vi "PSHet_zi_OptimizeModulation.vi"(0 "zi Address":string="DEV1925", 1 "Stop Program":bool=TRUE) -> ()   [LabVIEW 2022 SP3]
doc: "Control a Zurich instrument device via the LabOne Labview API. \nRequirements: Zurich Instruments MFLI, HF2 or UHFLI \nThis example polls demod data for a given time from the instrument.\n\n© Zurich Instruments AG, www.zhinst.com"
uses:
  PSHet_DAQInAndOut_control.ctl
  zi_OptimizeModulation_Control.ctl
  <vilib>/DAQmx/read.llb/DAQmx Read (Analog 2D DBL NChan NSamp).vi
  <vilib>/Analysis/baseanly.llb/Mean (DBL).vi
  <vilib>/DAQmx/write.llb/DAQmx Write (Analog 1D DBL NChan 1Samp).vi
  <vilib>/Analysis/1siggen.llb/Ramp Pattern by Samples.vi
  <vilib>/DAQmx/create/channels.llb/DAQmx Create Channel (AI-Voltage-Basic).vi
  <vilib>/DAQmx/configure/timing.llb/DAQmx Timing (Sample Clock).vi
  <vilib>/DAQmx/create/channels.llb/DAQmx Create Channel (AO-Voltage-Basic).vi
  <vilib>/DAQmx/miscellaneous.llb/DAQmx Fill In Error Info.vi
  <instrlib>/Zurich Instruments LabOne/Public/Configure/ziGetValueDouble.vi
  <instrlib>/Zurich Instruments LabOne/Public/Configure/ziSetValueDouble.vi
  <vilib>/addons/Time Series Analysis/Statistical Analysis.llb/TSA Deviation and Variance (Array).vi
  <vilib>/addons/Time Series Analysis/Statistical Analysis.llb/TSA Mean (Array).vi
  <instrlib>/Zurich Instruments LabOne/Zurich Instruments LabOne.lvlib
  <vilib>/Analysis/NI_AALBase.lvlib
  <vilib>/addons/_Advanced Signal Processing/NI_AdvSigProcTSA.lvlib
panel:
  out "Acquistion time (ms)":dbl
  out "PSHet running":bool
  out "PSHet input error":errorcluster={"status"=TRUE, "code"=-50103, "source"="DAQmx Control Task.vi:3900001<append>\n<B>Task Name: </B>_unnamedTask<1C21>"}
  out "Status":string="Running PSHet..."
  in  "Pause PSHet":bool
  in  "Enable PSHet":bool
  in  "Amplify amplitude by":dbl=1.0
  out "Amplitude / Re / Im":T1(graph)={"[0]"=nan, "[1]"=nan, "[2]"=nan, "[3]"=0.0, "[4]"=0.0, "[5]"=0.0, "[6]"=0.0, "[7]"=0.0, "[8]"=0.0}
  out "Phase (1 = pi radians)":dbl(graph)=nan
  in  "Phase offset (rad)":dbl
  in  "Channels to read":tag="Dev1/ai4:7"
  in  "Sampling rate":dbl=100000.0
  in  "Target acquistion time (ms)":dbl=1.0
  in  "DAQ Input range (V)":dbl=10.0
  in  "DAQ Output range (V)":dbl=10.0
  in  "Channels to output":tag="Dev1/ao0:1"
  out "Samples per loop":i32=100
  out "PSHet output error":errorcluster
  in  "Cancel Button":bool
  in  "Optimization order":i32=7
  in  "Slow wiggler amp":dbl=0.005
  out "Slow wiggler osc address":string="demods/4/oscselect/"
  out "Slow wiggler amp address":string="sigouts/0/amplitudes/4"
  out "Slow wiggler enable address":string="sigouts/0/enables/4"
  out "Fast wiggler amp address":string="sigouts/0/amplitudes/7"
  in  "Fast wiggler\nsource":i32=8
  in  "Slow wiggler oscillator":i32=6
  in  "Slow wiggler source":i32=5
  in  "Keep mod2 activated?":bool=TRUE
  in  "Optimize PSHet":bool
  out "Optimal modulation":dbl=0.27257525083612044
  out "Phase leakage vs. modulation amplitude":dbl[](graph)=[0.25054863863248045, 0.20185890824577868, 0.18656755567836747, 0.18956495717052135, 0.19995883483514376, 0.21035859208104846, 0.21622410115159774, 0.215277174673977, 0.20697395311525213, 0.1920364400403578, 0.1720414170679394, 0.14906497041965316, 0.12538086095847767, 0.1032109696116823, 0.08452605007414782, 0.07089502068789777, 0.06338102739261942, 0.06248250964430646, 0.06811750119592652, 0.0796493976371142, 0.09595242258818182, 0.1155150244432459, 0.1365794355592982, 0.15731562578657687, 0.17602788223479315, 0.19139224717292969, 0.2027230459557554, 0.21026673687437203, 0.21552131482737735, 0.22157950070474897]
  out "Chart length needed:":dbl=30000.0
  out "Samples per acquisition:":dbl=1000.0
  in  "Sample rate":dbl=1000.0
  out "Waveform Chart":dbl[][](graph)=[[-0.14092939771744095, -0.665227293227987, 0.6799915049443154], [-0.14651752916434696, -0.6540510435502394, 0.6702612579595977], [-0.15210566053411873, -0.6438609333196119, 0.6615837312250977], [-0.15605022380758304, -0.6346569625992535, 0.6535603510970559], [-0.15966607344125233, -0.6267678446953842, 0.6467852705127449], [-0.1616383550460539, -0.6198648664205069, 0.6405930146703966], [-0.1626244958448666, -0.6139480278180354, 0.6351211754543004], [-0.1636106366412881, -0.6083599024023401, 0.6299763577096781], [-0.16492549103279835, -0.6027717769195728, 0.62492738189584], [-0.16722648620771996, -0.596526224829899, 0.6195225860282997], [-0.16952748136963997, -0.5889658195561722, 0.6128787021466868], [-0.17380075806445489, -0.5814054141589, 0.6068269597810081], [-0.17906017547355835, -0.5722014422037289, 0.5995640390322362], [-0.18596316072028496, -0.5606964770008249, 0.5907307647873227], [-0.19450971372166492, -0.5498489381165337, 0.583239130614505], [-0.2037136936779682, -0.5383439723517474, 0.5755983856469543], [-0.21423252766169015, -0.5268390062961934, 0.5687309684406832], [-0.2250800749266365, -0.5150053266202999, 0.5620422818403096], [-0.23527019482571027, -0.5044864999816006, 0.5566495245996471], [-0.2454603144747226, -0.49495381312809744, 0.5524762828502897], [-0.25367815271970184, -0.48837954621470475, 0.5503337045176875], [-0.2602524231991969, -0.48279141926249386, 0.5484695782762677], [-0.2641969854372826, -0.4791755723738725, 0.5471830372681302], [-0.2651831259909967, -0.47818943230826244, 0.5467972416551268], [-0.26386827191886186, -0.4785181456637076, 0.5464486075148144], [-0.2609098502414599, -0.48049042579130036, 0.5467586297719736], [-0.2549930068238768, -0.4824627059101911, 0.5457029376164886], [-0.24743259566829118, -0.48312013261455505, 0.5427964185002083], [-0.2392147573001126, -0.4841062726692899, 0.5399838732294739], [-0.23165434585792594, -0.48279141926249386, 0.5354916343588915], [-0.22475136137733348, -0.4795042857285921, 0.5295635320460162], [-0.22014937165967374, -0.47424487202404514, 0.5228517423546106], [-0.21653352255986602, -0.4666844647151091, 0.514471725169238], [-0.21554738189078948, -0.4571517770555433, 0.5054190549484804], [-0.21686223611570166, -0.4463042356765767, 0.496202277540073], [-0.21982065810645296, -0.43414184048071797, 0.4866212689416064], [-0.22475136137733348, -0.42197944494915735, 0.47810022631302285], [-0.23033949168000983, -0.41080318929877785, 0.4709729734978992], [-0.23527019482571027, -0.3992982199486827, 0.46345564299888964], [-0.24052961144992746, -0.3914090979332085, 0.45940785357799563], [-0.24381674680628107, -0.38516354290282123, 0.4558481773624323], [-0.24578902800763247, -0.3818764086402205, 0.45413856670061553], [-0.24611774154028299, -0.38089026835658285, 0.45348797032516663], [-0.2431593197370876, -0.3818764086402205, 0.45272071550897236], [-0.23954347083795613, -0.3848348294776816, 0.45329782748234193], [-0.2332979135744604, -0.3900942442500595, 0.45453430659876654], [-0.22770978331166813, -0.3946962321236938, 0.4556718787334672], [-0.21982065810645296, -0.3992982199486827, 0.45580718531473446], [-0.2132463869871169, -0.40291406749137787, 0.45586595326423074], [-0.2073295428901606, -0.40521506136658475, 0.4551755543890379], [-0.2033849801116484, -0.4058724881858455, 0.4539800951596721], [-0.20042655800294967, -0.40357149431410305, 0.4506004396090042], [-0.19911170372558423, -0.3992982199486827, 0.44618890507798536], [-0.20075527157163386, -0.3940388052875831, 0.44223213263654454], [-0.2040424072440254, -0.3874645368718301, 0.4379064640847843], [-0.2093018242652489, -0.379904128070702, 0.4337446255181976], [-0.21554738189078948, -0.3749734266076287, 0.43251097616342704], [-0.22343650717751085, -0.37168629226770866, 0.4336756536853347], [-0.23198305940175373, -0.37102886539672636, 0.4375826308332858], [-0.24052961144992746, -0.3743159997416429, 0.4449347835883802], [-0.24644645507267404, -0.3815476952125904, 0.45421855855956317], [-0.2523632986113858, -0.39502494554137685, 0.4687557381899311], [-0.2569652879723781, -0.4127754697283867, 0.48622499692243043], [-0.2582801420662071, -0.4334844137038221, 0.5045962432578016], [-0.25795142854313763, -0.45780920379725293, 0.5254790258125629], [-0.25532172034927364, -0.4841062726692899, 0.5473098428859704], [-0.25104844449892694, -0.5104033399960459, 0.5688030335401263], [-0.24513160094155323, -0.5360429791639318, 0.5894332678862912], [-0.23822861668502254, -0.5600390504090917, 0.6086021785951613], [-0.2300107781348794, -0.579104421187336, 0.6231106552587046], [-0.22212165297351055, -0.5945539452051685, 0.634690808566435], [-0.21390381410376091, -0.6057301963011648, 0.6423892218890226], [-0.20601468863485567, -0.6113183217484084, 0.6450985525007843], [-0.19812556301479944, -0.6129618880436634, 0.6441863200301476], [-0.19220871870035822, -0.6119757482672057, 0.6414503160897497], [-0.18596316072028496, -0.6096747554473569, 0.6374053691136222], [-0.18070374340001494, -0.6073737626161406, 0.6336850403735805], [-0.17544432601207816, -0.605401483037473, 0.6303107703298462], [-0.17084233574204577, -0.606716336090847, 0.6303108884997144], [-0.16656905901621227, -0.6106608952286836, 0.6329707579209672], [-0.16196706864592386, -0.6188787266586344, 0.6397219783908993], [-0.15769379182687798, -0.6307124036639074, 0.6501272707064689], [-0.15177694692626514, -0.6445183597927491, 0.6621481388089782], [-0.14586010193930504, -0.660296594873264, 0.6762150268509062], [-0.1402719704833164, -0.6767322558564977, 0.691117046396554], [-0.13468383895005748, -0.6921817766633975, 0.705163348749226], [-0.12909570733940656, -0.7050015914223215, 0.7167237581952113], [-0.12482243017308409, -0.7142055607818862, 0.725031187002382], [-0.12153529386041878, -0.7188075453957481, 0.7290096809861984], [-0.12054915296137905, -0.7181501190250259, 0.7281975636703029], [-0.12054915296137905, -0.7119045684584879, 0.7220389275321463], [-0.12252143475703947, -0.700399606676483, 0.7110352389351007], [-0.12547985743239393, -0.6829778068812071, 0.6944090144241486], [-0.13172541634230234, -0.661282734548313, 0.6742747513604876], [-0.1396145432481224, -0.6359718155703369, 0.6511162499018224], [-0.14783238361122814, -0.6083599024023401, 0.6260640418480861], [-0.15769379182687798, -0.5800905610336973, 0.6011425712600368], [-0.16755519980307576, -0.552478644536341, 0.5773278077918655], [-0.1787314618874738, -0.5258528663350106, 0.5553973104914895], [-0.18957901008877137, -0.503171646634506, 0.537700573779793], [-0.198454276585324, -0.48312013261455505, 0.5222922193872981], [-0.2073295428901606, -0.46832803153231345, 0.5121686094187875], [-0.2125889598694254, -0.4581379171677425, 0.5050588252918282], [-0.21554738189078948, -0.4532072165848266, 0.5018540176231927], [-0.21521866833390724, -0.4525497898362953, 0.5011191350171089], [-0.2122602463101868, -0.4561656369411528, 0.5031316929886138], [-0.20667211576303285, -0.46241119096196653, 0.5064952842434298], [-0.198454276585324, -0.47128645178799705, 0.511365837276919], [-0.188264155776651, -0.48049042579130036, 0.5160566263767962], [-0.1777453211276332, -0.4900231129520875, 0.5212638970905425], [-0.16722648620771996, -0.497254806525035, 0.5246208538569838], [-0.15736507822355128, -0.5028429332971325, 0.5268916239713523], [-0.14881852444358756, -0.5054726399894023, 0.5269246084549691], [-0.1429016794133996, -0.5044864999816006, 0.524335311268329], [-0.14060068410051235, -0.49988451324996525, 0.5192813100398346], [-0.13994325686585313, -0.4916666796834451, 0.5111949129766116], [-0.1429016794133996, -0.4811478524985639, 0.5019204577850457], [-0.14881852444358756, -0.46701317807903536, 0.4901512641185856], [-0.1567076510160994, -0.4525497898362953, 0.4789139799252666], [-0.16656905901621227, -0.43710026096461424, 0.4677626423271532], [-0.17807403471451122, -0.42197944494915735, 0.45801420698391426], [-0.19056515082009318, -0.4075160552296692, 0.44987155053085504], [-0.20141269870821388, -0.39535365895881186, 0.44370214204243624], [-0.2132463869871169, -0.38516354290282123, 0.44025558070797083], [-0.22310779362690247, -0.3779318474922087, 0.43887306698627404], [-0.23033949168000983, -0.3723437191376913, 0.4378311622174617], [-0.23592762190737826, -0.370042725088378, 0.4388547153326528], [-0.23789990314613924, -0.3713575788323425, 0.44102473317622665], [-0.23625633544782199, -0.37365857287465826, 0.4420834594530314], [-0.2326404864886279, -0.3776031340615869, 0.44351518892457137], [-0.22672364266923783, -0.38319126234824924, 0.4452405570983544], [-0.21784837678163893, -0.3894368174069938, 0.44622746443768246], [-0.20634340219907543, -0.3956823723759986, 0.4462534475387141], [-0.194838427295084, -0.40094178701725985, 0.4457760977524653], [-0.1826760249030404, -0.4058724881858455, 0.4450876393931262], [-0.17215719011021052, -0.40948833567409954, 0.44420580270836985], [-0.1613096414459182, -0.41080318929877785, 0.44133894090761827], [-0.15309180135608064, -0.41080318929877785, 0.43840205289265827], [-0.14553138832638368, -0.41014576248693274, 0.43519987531500065], [-0.1402719704833164, -0.408830908860278, 0.4322255634998852], [-0.13665612067650917, -0.4078447686376922, 0.43013050417691295], [-0.1336976980832168, -0.4078447686376922, 0.429199755099981], [-0.13139670271787868, -0.41014576248693274, 0.4306792773876148], [-0.13041056184299937, -0.4154051769540436, 0.4353945057995416], [-0.128438280086001, -0.42296558513992805, 0.4420365120713579], [-0.1258085710616461, -0.4344705538687981, 0.45231897896466106], [-0.12252143475703947, -0.44794780256925676, 0.4644014812654556], [-0.11759073024973879, -0.46438347116082607, 0.47904027818967854], [-0.11134517112023401, -0.48180527920486077, 0.4945038667204414], [-0.10444218460072047, -0.5011993666066632, 0.5119657947666927], [-0.09655305700399536, -0.5202647398477764, 0.5291482706630452], [-0.08800650193159876, -0.5370291191029919, 0.544192446793202], [-0.08077480134248968, -0.5534647844398692, 0.5593280219575893], [-0.07452924163692604, -0.5662846029925139, 0.5711679783088023], [-0.06992725021203366, -0.575488575065966, 0.5797214161592379], [-0.06795496815643756, -0.5827202672803569, 0.5866692318474125], [-0.06795496815643756, -0.5853499735120398, 0.5892813158311471], [-0.07025596388701183, -0.586336113345062, 0.590530217918005], [-0.07518666897898041, -0.585021260233898, 0.5898329510275032], [-0.08274708333437564, -0.5833776938396811, 0.5892169494083235], [-0.09129363851958627, -0.5833776938396811, 0.5904778252431242], [-0.09984019352155787, -0.5833776938396811, 0.5918594410095414], [-0.1087154619839723, -0.586336113345062, 0.5963296818765454], [-0.117262016613767, -0.5925816655720455, 0.6040723556929807], [-0.12547985743239393, -0.6017856371215244, 0.6147285154171823], [-0.13139670271787868, -0.614605454333125, 0.6284941988444742], [-0.13599869343542947, -0.6300549771714588, 0.6445656823588045], [-0.1396145432481224, -0.6468193524415049, 0.6617155698479744], [-0.1402719704833164, -0.6645698667836539, 0.6792122890084631], [-0.14060068410051235, -0.6810055276190861, 0.6953683060201132], [-0.1396145432481224, -0.6954689086855423, 0.7093442208368523], [-0.13764226153612147, -0.7069738705856179, 0.720248183511481], [-0.13599869343542947, -0.7142055607818862, 0.7270386699948721], [-0.1336976980832168, -0.7181501190250259, 0.7304893345753994], [-0.132054129966458, -0.7178214058393291, 0.7298670179713213], [-0.13073927546822722, -0.7138768475935018, 0.7257498960936838], [-0.12975313459173926, -0.7073025837787141, 0.7191055701052711], [-0.12909570733940656, -0.6994134670823502, 0.7112277410152218], [-0.1287669937128379, -0.6908669238482197, 0.7027645730522731], [-0.12810956645889582, -0.6833065200907678, 0.6952120981519532], [-0.12745213920388054, -0.67771839549742, 0.6895986306419428], [-0.12613728469062985, -0.6760748294280814, 0.6877410774232803], [-0.12449371654302638, -0.677389682284006, 0.6887346855818444], [-0.12219272112510132, -0.6833065200907678, 0.6941461384280053], [-0.1198917256940083, -0.6925104898666277, 0.7028120690947217], [-0.11660458934101617, -0.7043441650327582, 0.7139309021684664], [-0.11397488023924437, -0.7191362585807737, 0.7281121010744867], [-0.1116738847610535, -0.7349144911993433, 0.7433507690938476], [-0.11003031655426035, -0.7497065838135313, 0.7577378388165568], [-0.10937288926965574, -0.7621976838940085, 0.7700050248151523], [-0.10970160291209288, -0.7710729390207922, 0.7788375433757959], [-0.1116738847610535, -0.7766610625368955, 0.7846486236517366], [-0.1152897347922843, -0.7766610625368955, 0.7851714010389163], [-0.1195630120599196, -0.7717303653200991, 0.7809373026113774], [-0.1258085710616461, -0.7605541181121651, 0.7708893326087386], [-0.13238284359034563, -0.7451045994928283, 0.7567734677315491], [-0.1402719704833164, -0.7250530958729975, 0.7384972698245339], [-0.14816109722228138, -0.7017144594655083, 0.7171853967790203], [-0.1567076510160994, -0.6764035426424031, 0.6943191199917923], [-0.16459677743531914, -0.6484629186123119, 0.6690263492249687], [-0.17380075806445489, -0.6221658591901174, 0.6459853402713998], [-0.17971760264493414, -0.5968549380998718, 0.6233251429508072], [-0.18760672861900846, -0.5735162953514401, 0.6034212671565087], [-0.19352357299982798, -0.5528073578377533, 0.5857024399694588], [-0.19812556301479944, -0.5360429791639318, 0.5714856203185472], [-0.20009784443400264, -0.5235518730839088, 0.560487030319885], [-0.20042655800294967, -0.5156627532770801, 0.5532439608980911], [-0.19812556301479944, -0.5110607666595257, 0.5481211963959736], [-0.194838427295084, -0.5110607666595257, 0.5469416056302939], [-0.18563444713974858, -0.5140191866333361, 0.5465124629796438], [-0.17610175318927423, -0.5189498865466406, 0.5480153394049361], [-0.16393935023956402, -0.526181579655643, 0.5511289915490549], [-0.15046209249218567, -0.5340706992793982, 0.554860660982478], [-0.1369848342966476, -0.5419598187662475, 0.5590038371822003], [-0.12317886202010969, -0.548205371596469, 0.5618737949894014], [-0.11003031655426035, -0.553793497740573, 0.5646183743917379], [-0.09885405256912966, -0.5564232041377004, 0.5651361834214876], [-0.09129363851958627, -0.5554370642405482, 0.5628897412160784], [-0.0866916472888084, -0.5518212179328075, 0.558589382525746], [-0.08570550630386592, -0.54491823853859, 0.5516170052697811], [-0.08833521559161803, -0.5347281259085266, 0.541975349025454], [-0.09392334777045852, -0.5215795931450926, 0.5299687417591823], [-0.10312733001207844, -0.5071162066642754, 0.5174959838075888], [-0.11397488023924437, -0.48969439960509303, 0.50278313250361], [-0.12646599831934513, -0.47161516514852736, 0.488277086016722], [-0.1402719704833164, -0.4525497898362953, 0.4737906056309553], [-0.15309180135608064, -0.43545669403156745, 0.46158382989371693], [-0.16854134058755144, -0.4186923109639196, 0.4513418158639376], [-0.18234731131986343, -0.40291406749137787, 0.4422559075106061], [-0.19319485942535564, -0.39042295767121954, 0.4356080113876762], [-0.2037136936779682, -0.3822051220676013, 0.4331050961679291], [-0.2122602463101868, -0.3766169937682243, 0.4323132801090846], [-0.21850580389095609, -0.3749734266076287, 0.43399292274863155], [-0.22179293942185763, -0.3779318474922087, 0.4382061037072189], [-0.22245036652490235, -0.3848348294776816, 0.44450198148734915], [-0.22047808521263307, -0.3946962321236938, 0.45210142856627855], [-0.21554738189078948, -0.4078447686376922, 0.46130036759697746], [-0.2089731107033897, -0.42263687174325054, 0.4714781928721327], [-0.20009784443400264, -0.4374289743504884, 0.4810231334857551], [-0.1902364372432495, -0.45189236308678876, 0.49030256971707475], [-0.18004631623022538, -0.4647121845264523, 0.49837143822195684], [-0.16919876777587567, -0.4755597254559905, 0.5047625931986757], [-0.1590086462375248, -0.48312013261455505, 0.5086146007693798], [-0.1498046652735464, -0.4867359794712938, 0.5092674655322084], [-0.14224425218248232, -0.4867359794712938, 0.5070950019383285], [-0.1369848342966476, -0.4821339925576467, 0.5012165516090394], [-0.13336898446040085, -0.47424487202404514, 0.4926413347021356], [-0.13304027083731707, -0.4627399043290507, 0.4814851324007063], [-0.1343551253280451, -0.44827651594706014, 0.4679777072164331], [-0.13895711601185873, -0.4301972798046227, 0.4520827132744958], [-0.14520267471319537, -0.41211804291950466, 0.4369497660414395], [-0.154735369387356, -0.38910810398508827, 0.4187459266981731], [-0.1655829182269603, -0.36642687727184187, 0.4021024237625902], [-0.17906017547355835, -0.34144465516461636, 0.3855476611018478], [-0.19319485942535564, -0.31744857203224575, 0.37161519020849354], [-0.2083156835788848, -0.29246634705880625, 0.35907100716551893], [-0.22409393427794427, -0.2668266935753615, 0.3484459438485796], [-0.23987218437553975, -0.2428306062021015, 0.3413288270064119], [-0.2569652879723781, -0.21883451744522248, 0.33751993311241724], [-0.2727435368257259, -0.19516714086823977, 0.3353792625594037], [-0.2878643580870167, -0.17281461729270303, 0.3357540477892614], [-0.3003554708937939, -0.1514482333181451, 0.3363777285597547], [-0.31284658333191384, -0.13238284359034563, 0.3397031085808872], [-0.32270798762880853, -0.1149610211544283, 0.3425733230482259], [-0.33125453783479286, -0.09885405256912966, 0.3456901684246783], [-0.33750009364637984, -0.08504807897921357, 0.3480509861347468], [-0.34144465516461636, -0.07321438694954918, 0.34920595498485146], [-0.3434169359101129, -0.06433911769566525, 0.34939192024966353], [-0.34210208208079046, -0.0577648440459419, 0.3469446811404721], [-0.3398010878697672, -0.05349156611494882, 0.3439856493560555], [-0.3358565263363857, -0.052505425047378484, 0.33993591446351945], [-0.3296109705007827, -0.05546384824269451, 0.33424486583395185], [-0.3220505606827909, -0.062038121930698104, 0.3279714807857356], [-0.31350401029215486, -0.07321438694954918, 0.3219396075751815], [-0.3039713192689968, -0.08932135657004811, 0.31682308577129925], [-0.2937812010415308, -0.11035903019615817, 0.3138256038490819], [-0.28293365556150724, -0.13599869343542947, 0.31392212101975475], [-0.2720861098020284, -0.1662403454200604, 0.31885216573293407], [-0.2602524231991969, -0.1987829901555856, 0.3274843522311402], [-0.25104844449892694, -0.23494148128448594, 0.34383545645188957], [-0.24052961144992746, -0.27307225033718857, 0.3638996398575702], [-0.2309969187694889, -0.31087430244508535, 0.38730144384150733], [-0.2214642258699434, -0.3467040704657786, 0.4114001893749113], [-0.21390381410376091, -0.3795754146415767, 0.4356975293577658], [-0.20601468863485567, -0.40850219545299654, 0.4575107601174367], [-0.20075527157163386, -0.43282698692594507, 0.4771183078390439], [-0.19681070873007078, -0.45090622296069977, 0.49198666341224845], [-0.19352357299982798, -0.46372604442884496, 0.5024870322587865], [-0.19286614585061995, -0.47030031170495185, 0.5083106662318306], [-0.19352357299982798, -0.47227259186886067, 0.5103849276155705], [-0.19516714086823977, -0.4696428849817093, 0.5085810184116454], [-0.19812556301479944, -0.46372604442884496, 0.5042772878105402], [-0.20174141227610976, -0.4568230636843234, 0.4993865325988384], [-0.20535726150562883, -0.4502487962087541, 0.4948692588356276], [-0.20995925138818072, -0.44400324201656344, 0.4911433254811718], [-0.21423252766169015, -0.44071610819576196, 0.4900267991972841], [-0.21686223611570166, -0.43841511450664145, 0.48911863804293315], [-0.21850580389095609, -0.4410448215789429, 0.49220455196557716], [-0.21883451744522248, -0.4456468089177948, 0.4964772143050443], [-0.21817709033642824, -0.4538646433323827, 0.5035815298587717], [-0.21653352255986602, -0.46241119096196653, 0.5105985467263379], [-0.2125889598694254, -0.47325873194754303, 0.5188139292877173], [-0.20765825645333097, -0.48279141926249386, 0.5255563775530943], [-0.20174141227610976, -0.49068053964535335, 0.5305346260271939], [-0.19549585444113232, -0.4975835198664926, 0.5346101274259557], [-0.18925029651113684, -0.5002132265895001, 0.5348167413092374], [-0.18234731131986343, -0.5002132265895001, 0.5324131985597856], [-0.17610175318927423, -0.4975835198664926, 0.5278268529727], [-0.17084233574204577, -0.4913379663376554, 0.5201923690776528], [-0.1655829182269603, -0.4824627059101911, 0.5100862333005467], [-0.16098092784551665, -0.4735874453066194, 0.5001998875270302], [-0.1567076510160994, -0.46339733106248987, 0.48917724223723086], [-0.15177694692626514, -0.4532072165848266, 0.477946673576482], [-0.14684624277646752, -0.44498938215803535, 0.4685929675645541], [-0.14191553856662292, -0.43775768773611773, 0.46018671564781943], [-0.1363274070561032, -0.4318408467572898, 0.4528484060286549], [-0.12975313459173926, -0.4265814324871455, 0.44587845258452113], [-0.1241650029127001, -0.4232942985363594, 0.44112924537112636], [-0.11824815752087511, -0.4200071645609699, 0.4363354730475479], [-0.11298873932163633, -0.41672003056095214, 0.431766185665591], [-0.1087154619839723, -0.4131041831324574, 0.42716989336319505], [-0.1060857528304466, -0.4078447686376922, 0.4214161153287037], [-0.10444218460072047, -0.40159921384295644, 0.4149579478494798], [-0.10509961189342096, -0.39502494554137685, 0.4087672149526127], [-0.10542832553936615, -0.3868071100247859, 0.40091753789496587], [-0.10772932105342398, -0.37826056092258104, 0.3933022483588129], [-0.1106877438377864, -0.3697140116517618, 0.38592774848090217], [-0.11331745296110843, -0.3614961756550187, 0.37884077151066664], [-0.11594716206718864, -0.35525062019272474, 0.3736933870685304], [-0.117262016613767, -0.3499912049962634, 0.3691127525771276], [-0.11791944388544148, -0.3463753570113456, 0.36589736701838793], [-0.11660458934101617, -0.3434169359101129, 0.3626731615728928], [-0.11430359387790834, -0.3434169359101129, 0.36193991689684685], [-0.10937288926965574, -0.3440743628232617, 0.36103960455804], [-0.10641446647558184, -0.3453892166465354, 0.36141077688828], [-0.10148376177019686, -0.3473614973738892, 0.3618825275705647], [-0.09622434335075086, -0.34834763773416705, 0.36139341577878487], [-0.09227977949069568, -0.3486763511870896, 0.36068096093361246], [-0.08997878388764544, -0.3490050646397605, 0.3604174200758102], [-0.08932135657004811, -0.3476902108275669, 0.35898020480916715], [-0.09096492486200772, -0.34473178973540247, 0.3565313792772306], [-0.09589562969723567, -0.34111594170615106, 0.35433890201486995], [-0.10312733001207844, -0.3358565263363857, 0.3513329652596856], [-0.11266002568189482, -0.33026839743514586, 0.34895486202519754], [-0.1258085710616461, -0.32468026846077536, 0.34820263250058064], [-0.13994325686585313, -0.3187634259374788, 0.34812962651521157], [-0.15572151020292557, -0.31350401029215486, 0.3500485012239638], [-0.1741294716545091, -0.3089020215490944, 0.354600524274564], [-0.19155129154904277, -0.306601027158851, 0.3615191380120406], [-0.2089731107033897, -0.30725845412876585, 0.37158783434155923], [-0.2250800749266365, -0.3102168754807733, 0.38326955261543266], [-0.24020089791286348, -0.31679114507810524, 0.39755892765481066], [-0.2523632986113858, -0.32698126275320416, 0.4130423473176805], [-0.26189599080291753, -0.34111594170615106, 0.43005766553418867], [-0.26847026115328043, -0.3582090412124717, 0.44764941453113605], [-0.27307225033718857, -0.37727442063071553, 0.4657300101630324], [-0.27307225033718857, -0.3986407931195172, 0.48320072003586034], [-0.2710999692645514, -0.42165073155174165, 0.5012828869544218], [-0.2671554070914608, -0.4420309617270178, 0.516491415866243], [-0.2609098502414599, -0.461753764227069, 0.5303682576577228], [-0.2533494391930111, -0.47687457888406243, 0.5399956502836528], [-0.24480288740812445, -0.4929815330641953, 0.5504173376863043], [-0.23559890836667435, -0.502185506621665, 0.5547045417917784], [-0.22573750202445986, -0.5090884866662126, 0.5568918270870363], [-0.217519663226588, -0.5123756199836123, 0.556635949111984], [-0.20634340219907543, -0.5150053266202999, 0.5548045476367071], [-0.1974681358729612, -0.5153340399488096, 0.5518721205271231], [-0.1885928693550767, -0.5182924598946399, 0.5515381621929872], [-0.18004631623022538, -0.5225657331155742, 0.5527129647608168], [-0.17084233574204577, -0.5294687128488675, 0.5563490105748679], [-0.1616383550460539, -0.5413023921475639, 0.564920558633397], [-0.15309180135608064, -0.5560944908388858, 0.5767826127613499], [-0.1429016794133996, -0.575488575065966, 0.5929654205859107], [-0.1336976980832168, -0.598169791177434, 0.6129291749868054], [-0.12383628928210527, -0.6234807121962402, 0.6356599916810025], [-0.11331745296110843, -0.6487916318457858, 0.6586132603422973], [-0.10279861636424256, -0.6760748294280814, 0.6838455458015443], [-0.09326592045936613, -0.6997421802806196, 0.7059303441438171], [-0.08373322432665023, -0.7201223981345077, 0.724974152057252], [-0.07715895099860967, -0.7355719175473041, 0.7396076997999844], [-0.07058467756171738, -0.7470768784927337, 0.7504039306166636], [-0.0672975408023899, -0.7520075759576037, 0.7550128166433205], [-0.06565397241249496, -0.7510214364686147, 0.753885695665412], [-0.06598268609101984, -0.744775886325401, 0.7476930090054158], [-0.06894110918546298, -0.7335996385007506, 0.7368319388735493], [-0.07452924163692604, -0.7194649717655752, 0.7233149061485014], [-0.08208965600483406, -0.7036867386422951, 0.7084587057578033], [-0.08997878388764544, -0.6859362257591042, 0.6918126100025529], [-0.09786791161426697, -0.6695005650939518, 0.6766159433422027], [-0.10838674834072598, -0.6550371832383053, 0.6639438219011071], [-0.117262016613767, -0.6432035068455573, 0.6538051175684925], [-0.12515114380287323, -0.6339995361123312, 0.6462338745267217], [-0.131067989093187, -0.6303836904177982, 0.6438652148623143], [-0.13599869343542947, -0.6287401241837955, 0.6432804896581261], [-0.13895711601185873, -0.6300549771714588, 0.6451963688280186], [-0.13994325686585313, -0.6346569625992535, 0.6499027429684633], [-0.14060068410051235, -0.6382728082608786, 0.6535753438852787], [-0.14060068410051235, -0.642874793608186, 0.6580703249853315], [-0.1396145432481224, -0.6455044995007344, 0.6604303744998979], [-0.1396145432481224, -0.6468193524415049, 0.6617155698479744], [-0.1392858296301243, -0.6445183597927491, 0.6593970415809337], [-0.14092939771744095, -0.6402450877009507, 0.6555721680076105], [-0.14454524748601766, -0.6330133963802218, 0.6493067753901987], [-0.14881852444358756, -0.6228232856936409, 0.6403559935065724], [-0.15407794217564486, -0.6113183217484084, 0.6304364383269513], [-0.16065221424484938, -0.598169791177434, 0.619367607337539], [-0.16788391339816627, -0.5846925469555224, 0.608317666062082], [-0.17544432601207816, -0.5718727289162142, 0.5981798472097754], [-0.18201859773642226, -0.5593816238164158, 0.5882504322016462], [-0.1885928693550767, -0.548534084900955, 0.580049060571353], [-0.19352357299982798, -0.5393301122858216, 0.5729994269847543], [-0.19615328158612783, -0.5320984193863076, 0.5671021405270956], [-0.19681070873007078, -0.526181579655643, 0.5617842199988716], [-0.19615328158612783, -0.522237019792319, 0.5578598522196858], [-0.19319485942535564, -0.5179637465682814, 0.5528206729740067], [-0.18957901008877137, -0.5156627532770801, 0.5494072043425872], [-0.18563444713974858, -0.5113894799909064, 0.5440398406461147], [-0.18070374340001494, -0.5081023466663224, 0.5392789978912604], [-0.1770878939530834, -0.5025142199595187, 0.5328045264881504], [-0.1744581852442985, -0.4942963864410928, 0.5241799080921131], [-0.17380075806445489, -0.4854211260722226, 0.5155971035033108], [-0.17478689883382315, -0.4739161586654533, 0.5051207632320851], [-0.17807403471451122, -0.4601101973855695, 0.49336776909086055], [-0.18300473848595328, -0.4463042356765767, 0.4823672927253313], [-0.18957901008877137, -0.4321695601470869, 0.4719223768629382], [-0.19516714086823977, -0.41672003056095214, 0.4601584474345812], [-0.20108398514005532, -0.40390020772509433, 0.4511874852876355], [-0.2073295428901606, -0.39272395161238255, 0.4440919291375243], [-0.21160281919092377, -0.38450611605229307, 0.43888575548901815], [-0.21390381410376091, -0.3795754146415767, 0.4356975293577658], [-0.21521866833390724, -0.3776031340615869, 0.43462995991136316], [-0.2145612412193576, -0.3776031340615869, 0.43430479284337187], [-0.21193153275068627, -0.38089026835658285, 0.4358811433209802], [-0.2102879649492535, -0.38549225632771184, 0.4391187856276804], [-0.20700082932672786, -0.39042295767121954, 0.44190432133969454], [-0.20437112080982006, -0.39535365895881186, 0.44505288525430614], [-0.20305626654506598, -0.3992982199486827, 0.4479630741896116], [-0.2033849801116484, -0.40225664066766237, 0.45075032456588254], [-0.2040424072440254, -0.40422892113583814, 0.4528071605403125], [-0.20667211576303285, -0.40422892113583814, 0.4539982203892567], [-0.2109453920706127, -0.40521506136658475, 0.45683389146838654], [-0.21521866833390724, -0.40521506136658475, 0.4588227557104654], [-0.21949194455297083, -0.4065299150041169, 0.46199922674924354], [-0.22442264782776938, -0.40915962226731223, 0.4666659633527569], [-0.22770978331166813, -0.4134328965362813, 0.4719941793647739], [-0.22968206458948842, -0.41902102436355165, 0.47784146916395825], [-0.23033949168000983, -0.4269101458808718, 0.48508613058242817], [-0.22968206458948842, -0.43578540741866695, 0.4926081324066255], [-0.2270523562169754, -0.4453180955380373, 0.4998609593450011], [-0.22343650717751085, -0.4558369235692022, 0.5076526111709863], [-0.21982065810645296, -0.4647121845264523, 0.5140802818409801], [-0.2145612412193576, -0.47293001858822453, 0.5193258406005326], [-0.2106166785100641, -0.4795042857285921, 0.5237210567646665], [-0.20700082932672786, -0.48312013261455505, 0.5255990923502992], [-0.20469983437535216, -0.4841062726692899, 0.5256052753074777], [-0.20272755297822093, -0.4811478524985639, 0.5221127432849318], [-0.20272755297822093, -0.47588843881337156, 0.5172700135642558], [-0.20469983437535216, -0.4666844647151091, 0.5096041716859513], [-0.20700082932672786, -0.4561656369411528, 0.5009355564020992], [-0.21160281919092377, -0.4426883884911778, 0.4906615558554213], [-0.21653352255986602, -0.42986856641335275, 0.48132499496956843], [-0.22245036652490235, -0.41737745736292714, 0.4729567712611856], [-0.2290246374979244, -0.40521506136658475, 0.46545840903283797], [-0.23461276774300144, -0.3973259394582111, 0.4614228569916986], [-0.23954347083795613, -0.3933813784504793, 0.46057570857861574], [-0.2428306062021015, -0.3946962321236938, 0.46341322700277005], [-0.2444741738744362, -0.39962693336289373, 0.46847551436613927], [-0.24348803327181412, -0.4114606161096351, 0.47810695556109256], [-0.24085832498673154, -0.4265814324871455, 0.48988207893144964], [-0.23559890836667435, -0.4456468089177948, 0.5040911861183274], [-0.2290246374979244, -0.4653696112569759, 0.5186724974996502], [-0.2208067987653311, -0.4867359794712938, 0.5344787704791213], [-0.2122602463101868, -0.5054726399894023, 0.5482307925878636], [-0.2033849801116484, -0.5225657331155742, 0.5607498511472233], [-0.19385228657403697, -0.5367004057902094, 0.5706365170450959], [-0.1853057335589483, -0.5452469518454433, 0.5758753800837183], [-0.1777453211276332, -0.550506364722904, 0.5784899798468358], [-0.17084233574204577, -0.5514925046306862, 0.5773483232379093], [-0.16492549103279835, -0.550506364722904, 0.5746804983578586], [-0.15999478704271725, -0.5459043784584396, 0.5688672273043507], [-0.1567076510160994, -0.5409736788378665, 0.5632138218140236], [-0.15374922856938977, -0.5370291191029919, 0.5586046008136863], [-0.1511195197097585, -0.5350568392227344, 0.5559882466710345], [-0.14816109722228138, -0.5350568392227344, 0.555191437190032], [-0.14520267471319537, -0.5393301122858216, 0.5585344991691229], [-0.14092939771744095, -0.5465618050704886, 0.5644385723025238], [-0.13599869343542947, -0.5583954839256335, 0.5747183319546075], [-0.1300818482175034, -0.5731875820648644, 0.5877629551690438], [-0.12383628928210527, -0.5896232461066138, 0.6024873433462828], [-0.11660458934101617, -0.6103321819684733, 0.6213710667562375], [-0.1087154619839723, -0.6307124036639074, 0.6400134278356135], [-0.10279861636424256, -0.6501064847773921, 0.6581838626675833], [-0.09688177065696921, -0.6671995725555206, 0.6741968162961756], [-0.09195106583393023, -0.6826490936714198, 0.6888140413772114], [-0.08997878388764544, -0.6931679162724105, 0.6989835060281001], [-0.09030749754603731, -0.6984273274861903, 0.7042415607535029], [-0.09326592045936613, -0.6990847538838554, 0.7052786860752163], [-0.09951147987101891, -0.6934966294749632, 0.7005998213811181], [-0.10937288926965574, -0.6842926597180914, 0.692978263043836], [-0.12054915296137905, -0.670486704749867, 0.6812374912804208], [-0.13468383895005748, -0.653064903860116, 0.6668084471031749], [-0.15013337888299938, -0.6323559698909977, 0.6499339228810962], [-0.1655829182269603, -0.6113183217484084, 0.633346503356454], [-0.18037502981525233, -0.5896232461066138, 0.6165960782636828], [-0.19450971372166492, -0.567270742866339, 0.5996916911582252], [-0.20535726150562883, -0.5475479449867868, 0.5847908659617937], [-0.21291767342840207, -0.5288112862121277, 0.5700660594031963], [-0.21916323099922735, -0.5110607666595257, 0.5560716042387372], [-0.22179293942185763, -0.4959399531567997, 0.5432757542119439], [-0.22212165297351055, -0.48180527920486077, 0.5305415683896583], [-0.2211355123177679, -0.46832803153231345, 0.5179112471524182], [-0.21982065810645296, -0.4558369235692022, 0.5060715587932094], [-0.21883451744522248, -0.4423596751092201, 0.4935287511262319], [-0.21784837678163893, -0.42986856641335275, 0.4819179387164022], [-0.2171909496712756, -0.4163913171595948, 0.46963138483816524], [-0.21850580389095609, -0.40225664066766237, 0.4577719861407705], [-0.22212165297351055, -0.38812196371787927, 0.4471875305058354], [-0.22606621557298007, -0.3730011460066744, 0.4361602787345284], [-0.23132563231383774, -0.3588664681029879, 0.42696216471030507], [-0.23757118960699586, -0.3450605031910949, 0.4189353422591305], [-0.24381674680628107, -0.33191196476662593, 0.41183996695129055], [-0.24907616332246757, -0.3204069933133073, 0.40583195598611294], [-0.2540068662461338, -0.31153172940837925, 0.40195958320253655], [-0.2569652879723781, -0.3036426057816176, 0.3977813359982819], [-0.25795142854313763, -0.29969804391316635, 0.39542111351421744], [-0.2549930068238768, -0.2973970494729249, 0.3917479273260843], [-0.24973359038232373, -0.29904061693151734, 0.3896051292527201], [-0.24151575205956038, -0.30134161136282056, 0.3861821140752588], [-0.23033949168000983, -0.3069297406439358, 0.38374750438166894], [-0.21817709033642824, -0.31284658333191384, 0.3814108381392984], [-0.2040424072440254, -0.3197495663637374, 0.3793060626245444], [-0.19089386439667327, -0.32599512234368355, 0.3777741220043648], [-0.17741660754049055, -0.3309258243684969, 0.37548442559598355], [-0.16459677743531914, -0.3351990994106198, 0.373430763847574], [-0.1544066557816336, -0.33651395326114103, 0.37024729045478416], [-0.14553138832638368, -0.3355278128736291, 0.36572981584766334], [-0.1382996887745252, -0.33289810516247864, 0.3604829431968997], [-0.13402641170576485, -0.32698126275320416, 0.35338339693087323], [-0.13139670271787868, -0.3204069933133073, 0.34630295241190817], [-0.13041056184299937, -0.31284658333191384, 0.3389393741403599], [-0.12975313459173926, -0.30594360018791694, 0.3323211736142101], [-0.13041056184299937, -0.30068418438372474, 0.3277466908737791], [-0.13139670271787868, -0.2973970494729249, 0.3251308944415032], [-0.13271155721396527, -0.29805447645712824, 0.3262649664832073], [-0.132054129966458, -0.30134161136282056, 0.32900617012442085], [-0.13139670271787868, -0.3089020215490944, 0.3356866878537899], [-0.12975313459173926, -0.3187634259374788, 0.344159843171426], [-0.12810956645889582, -0.3355278128736291, 0.35915313479078437], [-0.1241650029127001, -0.35360705295074235, 0.3747731258305749], [-0.1198917256940083, -0.3730011460066744, 0.391795713111029], [-0.11627587570423698, -0.3946962321236938, 0.4114671249607044], [-0.11266002568189482, -0.4163913171595948, 0.43136296826749915], [-0.11003031655426035, -0.43677154757849485, 0.45041764545268886], [-0.10772932105342398, -0.4558369235692022, 0.4683939661264504], [-0.10740060740936822, -0.4739161586654533, 0.48593355092658536], [-0.10772932105342398, -0.48969439960509303, 0.5014042397300049], [-0.10970160291209288, -0.5038290733085331, 0.5156337622697119], [-0.11298873932163633, -0.516320179932904, 0.5285385354157623], [-0.117262016613767, -0.5284825728934006, 0.5413355802017413], [-0.12153529386041878, -0.540644965527932, 0.5541369924526218], [-0.12679471194779196, -0.5531360711389295, 0.567482521469106], [-0.131067989093187, -0.5669420295752992, 0.5818952505940319], [-0.13501255257180217, -0.5817341274396153, 0.5971959346645657], [-0.1382996887745252, -0.5984985044462423, 0.6142696995127785], [-0.13994325686585313, -0.6169064471286443, 0.6325801764607463], [-0.14060068410051235, -0.635643102327911, 0.6510074545706702], [-0.1402719704833164, -0.6543797567798233, 0.6692451656803305], [-0.1386284023933257, -0.6734451237053358, 0.6875653922301652], [-0.13501255257180217, -0.6905382106438607, 0.7036131108152964], [-0.13238284359034563, -0.7050015914223215, 0.7173231218809777], [-0.12909570733940656, -0.7165065530943033, 0.7280435030137563], [-0.1258085710616461, -0.7247243826919954, 0.7355632042325574], [-0.12285014838870895, -0.7286689408492888, 0.7389523559185343], [-0.12120658022767436, -0.7289976540276133, 0.7390051519903305], [-0.11890558479093533, -0.7263679485947732, 0.7360359602901568], [-0.11824815752087511, -0.7214372508696887, 0.7310638369523524], [-0.11759073024973879, -0.7145342739700464, 0.7241455713588036], [-0.117262016613767, -0.7076312969715859, 0.7172812788537117], [-0.11791944388544148, -0.7013857462685895, 0.7112291897236769], [-0.11759073024973879, -0.6977699010876239, 0.7076089419336781], [-0.117262016613767, -0.6954689086855423, 0.7052853206246296], [-0.1156184484298711, -0.6977699010876239, 0.7072838613181862], [-0.11298873932163633, -0.7030293122509328, 0.7120510298409183], [-0.10904417562694887, -0.7115758552685341, 0.7198825112747959], [-0.10279861636424256, -0.7240669563293214, 0.7313279105670795], [-0.09523820238939307, -0.7365580570675769, 0.7426897647238225], [-0.0866916472888084, -0.7500352969776343, 0.7550287335075236], [-0.07551538264959917, -0.764169962824945, 0.7678921181393863], [-0.06401040401577515, -0.7746887836561054, 0.7773287871582004], [-0.052176711357640404, -0.7832353254158497, 0.7849713269842221], [-0.04132915944241505, -0.7875085962402038, 0.7885923462552961], [-0.031139034643375835, -0.7881660225175937, 0.7887809065448563], [-0.022921191870621138, -0.784550177981127, 0.7848849360301088], [-0.016675631247889122, -0.7773184888287366, 0.7774973374568599], [-0.01273106659260495, -0.7664709549010125, 0.7665766789848588], [-0.010758784250008285, -0.7536511417681602, 0.7537279316351423], [-0.011087497974467092, -0.7405026151286573, 0.7405856166735311], [-0.013059780315401476, -0.7273540881337612, 0.7274713240992953], [-0.015032062646365224, -0.7145342739700464, 0.7146923754912359], [-0.01799048612412768, -0.7036867386422951, 0.7039166738556576], [-0.020948909579486336, -0.6941540558793919, 0.6944700930251637], [-0.022592478156122725, -0.686264938966628, 0.6866367209260691], [-0.02456476043897063, -0.6800193879849667, 0.6804629273449603], [-0.023907333012459286, -0.6750886897837547, 0.6755118797221225], [-0.023578619298789433, -0.670486704749867, 0.6709011645051547], [-0.022921191870621138, -0.665556006449812, 0.6659505828199207], [-0.022592478156122725, -0.6606253080985085, 0.6610115110718452], [-0.022592478156122725, -0.653064903860116, 0.6534555751717613], [-0.02522218786437755, -0.6435322200826994, 0.6440263015166646], [-0.028838038684383893, -0.6313698301554347, 0.6320280807888716], [-0.03574102652085526, -0.6169064471286443, 0.6179409239447176], [-0.04363015532819994, -0.6004707840542041, 0.6020537791232885], [-0.05447770718005396, -0.5820628407200967, 0.5846066807065622], [-0.0672975408023899, -0.5633261833583318, 0.5673317793453089], [-0.08241836966974073, -0.5409736788378665, 0.5472159618052028], [-0.09819662526615838, -0.5199360265228508, 0.5291276300572791], [-0.11266002568189482, -0.5008706532678491, 0.5133845466038174], [-0.12745213920388054, -0.4814765658518331, 0.49805996752612025], [-0.14060068410051235, -0.4656983246218734, 0.48646015450923813], [-0.1511195197097585, -0.4525497898362953, 0.47711468382159766], [-0.15933735983952152, -0.4433458152543596, 0.4711092295255761], [-0.16393935023956402, -0.4361141208055213, 0.46590947288388895], [-0.16656905901621227, -0.4321695601470869, 0.463158482745672], [-0.16656905901621227, -0.42921113963007645, 0.46039923306201913], [-0.16328192304274658, -0.42953985302183745, 0.45952744393187134], [-0.15933735983952152, -0.42986856641335275, 0.4584488833347729], [-0.15374922856938977, -0.42953985302183745, 0.45622725764656386], [-0.14816109722228138, -0.42921113963007645, 0.4540637764815195], [-0.1429016794133996, -0.42625271909317336, 0.4495689830420842], [-0.13895711601185873, -0.422308158346327, 0.4445821191818218], [-0.13534126619327902, -0.41507646355169997, 0.4365841601906621], [-0.1336976980832168, -0.4058724881858455, 0.427326047812347], [-0.13304027083731707, -0.3940388052875831, 0.4158921659961059], [-0.13402641170576485, -0.3792467012122018, 0.4022326931206118], [-0.13566997981448808, -0.3637971697498838, 0.38827145676818603], [-0.13764226153612147, -0.34933377809217975, 0.37547234342483116], [-0.1392858296301243, -0.3332268186272572, 0.3611656891070842], [-0.1392858296301243, -0.3194208528885718, 0.34846839683939007], [-0.13895711601185873, -0.307587167613341, 0.3375188080251687], [-0.13599869343542947, -0.29871190344030973, 0.3282140244917588], [-0.13172541634230234, -0.29509605502016273, 0.32316136371635734], [-0.12646599831934513, -0.2941099145365725, 0.32014729509964407], [-0.1195630120599196, -0.29673962248769936, 0.3199214238011934], [-0.11134517112023401, -0.3026564653179497, 0.322488268206069], [-0.10378475730693973, -0.31087430244508535, 0.3277409156177769], [-0.09622434335075086, -0.3200782798386492, 0.334229306730801], [-0.08965007022898236, -0.32895354356540724, 0.3409509772918971], [-0.08406193799019845, -0.33782880710762103, 0.3481303094107524], [-0.07978866034287696, -0.3450605031910949, 0.3541651891163255], [-0.07748766466759524, -0.3509773453505023, 0.35942931867743266], [-0.07584409631994568, -0.3545931932966854, 0.36261365070682283], [-0.07485795530808936, -0.3582090412124717, 0.3659473058778629], [-0.07485795530808936, -0.3611674622118925, 0.36884366503098126], [-0.07518666897898041, -0.3637971697498838, 0.3714854181662862], [-0.07485795530808936, -0.36839915790279604, 0.3759277231282593], [-0.07321438694954918, -0.3756308534726159, 0.3826994702595813], [-0.07091339123615026, -0.3848348294776816, 0.39131388300918685], [-0.06631139976927175, -0.3976546528739095, 0.40314566187871803], [-0.06006583983578334, -0.4131041831324574, 0.4174481659280741], [-0.05184799766762835, -0.4324982735366388, 0.43559496263652503], [-0.04198658683972736, -0.45353592995872644, 0.4554752608407802], [-0.029495466102617218, -0.4762171521705106, 0.47712970829953766], [-0.016346917528137828, -0.4979122332077099, 0.49818050312167034], [-0.002212227316732457, -0.5192785998722829, 0.5192833121091216], [0.011265035921287303, -0.539658825596705, 0.5397763880337141], [0.023427444611510473, -0.5570806307346219, 0.5575730214964759], [0.03460371239416328, -0.570886589052261, 0.5719343620304546], [0.040849273943313294, -0.5820628407200967, 0.5834944847458667], [0.04643740804696267, -0.5889658195561722, 0.5907936775826175], [0.04775226314199056, -0.5942252319335644, 0.5961408431752351], [0.04676612182029741, -0.5968549380998718, 0.598684296841259], [0.0428215565588506, -0.5994846442512705, 0.6010120834053132], [0.036575994977682005, -0.600799497321383, 0.6019118202778826], [0.02901557846235757, -0.6040866299803822, 0.6047830688061302], [0.019154165838942444, -0.6086886156639422, 0.6089899119918752], [0.008306612243586142, -0.6142767410756962, 0.6143329019623995], [-0.0028696547797994465, -0.6218371459380092, 0.6218437673458537], [-0.013388494037921028, -0.6293975506780882, 0.6295399340567523], [-0.023907333012459286, -0.6379440950200623, 0.6383919085818169], [-0.03311131688319169, -0.6464906392066561, 0.6473380151725757], [-0.042315300537971334, -0.653064903860116, 0.6544343766287353], [-0.04987571552180023, -0.6573381758357935, 0.659227627159193], [-0.05710741667495384, -0.6599678816477914, 0.6624340433929705], [-0.06269554929348325, -0.6593104551961617, 0.6622846882060475], [-0.0672975408023899, -0.6550371832383053, 0.6584851330309762], [-0.07058467756171738, -0.6484629186123119, 0.6522931499883234], [-0.07255695960422626, -0.6392589479819486, 0.6433634392487632], [-0.07354310062180197, -0.6284114109363035, 0.6327001572972969], [-0.07485795530808936, -0.6165777338728362, 0.621105317462884], [-0.07551538264959917, -0.6034292034504425, 0.6081359852808834], [-0.07551538264959917, -0.5915955257523353, 0.5963957068146093], [-0.07650152365982202, -0.5804192743153491, 0.5854391660275479], [-0.07683023732935193, -0.5702291624751175, 0.5753817716135596], [-0.07683023732935193, -0.5623400434760335, 0.5675642781788789], [-0.07781637833630875, -0.555765777539835, 0.5611871240698925], [-0.07847380567291956, -0.548534084900955, 0.5541189226825947], [-0.08077480134248968, -0.5432746720007695, 0.549246700280905], [-0.08241836966974073, -0.5376865457278444, 0.5439665514677895], [-0.0853767926416755, -0.5311122794365519, 0.5379307112352572], [-0.08965007022898236, -0.5235518730839088, 0.5311720050056581], [-0.09425206142559839, -0.5156627532770801, 0.5242056144303241], [-0.09951147987101891, -0.5058013533248564, 0.5154973750189], [-0.10509961189342096, -0.49528252647123877, 0.5063108822135676], [-0.1106877438377864, -0.48476369937123903, 0.49724000328210566], [-0.1156184484298711, -0.47325873194754303, 0.4871770242754959], [-0.12054915296137905, -0.4627399043290507, 0.47818439679496544], [-0.12383628928210527, -0.45189236308678876, 0.46855323535253], [-0.12613728469062985, -0.44301710187289106, 0.46062432321902036], [-0.12646599831934513, -0.4344705538687981, 0.45250227724285413], [-0.12613728469062985, -0.42789628606057645, 0.44610071308344673], [-0.1241650029127001, -0.4213220181540797, 0.43923705550617825], [-0.12252143475703947, -0.41672003056095214, 0.43435824597403966], [-0.12022043932782811, -0.41080318929877785, 0.42803295944380676], [-0.11824815752087511, -0.40521506136658475, 0.4221159470043826], [-0.11791944388544148, -0.3986407931195172, 0.4157156205691693], [-0.11890558479093533, -0.39272395161238255, 0.4103299163655013], [-0.12186400749289447, -0.38450611605229307, 0.403355661425308], [-0.12712342557597045, -0.3746447131747607, 0.39562485569029665], [-0.13402641170576485, -0.3641258831910051, 0.3880086826919633], [-0.14224425218248232, -0.3526209126025377, 0.38023010833388793], [-0.15342051496286835, -0.34144465516461636, 0.37432914253629185], [-0.1642680638375743, -0.3292822570332215, 0.367982066945983], [-0.17511561242308304, -0.317777285508935, 0.36283313092899694], [-0.18464830639655566, -0.3085733080655381, 0.35960044981288025], [-0.19220871870035822, -0.2993693304224695, 0.3557614194119862], [-0.19812556301479944, -0.29213763356248545, 0.352984611085838], [-0.20272755297822093, -0.28885049858519735, 0.352892435834851], [-0.20469983437535216, -0.28490593657863494, 0.35081820775302663], [-0.20437112080982006, -0.28293365556150724, 0.34902579914736914], [-0.2033849801116484, -0.28096137453514125, 0.3468497428508367], [-0.20108398514005532, -0.2799752340184922, 0.34470407706250805], [-0.19779684944401188, -0.27833166648560687, 0.341455868625262], [-0.19648199515823084, -0.27570195841962686, 0.33855094786128825], [-0.19418100014798262, -0.27241482331400585, 0.33453863271627066], [-0.19385228657403697, -0.26847026115328043, 0.33114194861674223], [-0.19319485942535564, -0.2628821313620513, 0.3262380552569515], [-0.19418100014798262, -0.25795142854313763, 0.3228702530520832], [-0.1958245680137617, -0.2530207256660615, 0.31994804117912135], [-0.1974681358729612, -0.24907616332246757, 0.31785625653836486], [-0.1987829901555856, -0.24743259566829118, 0.31739181869472266], [-0.198454276585324, -0.2487474497921507, 0.31821281192482304], [-0.1974681358729612, -0.2530207256660615, 0.32095662059182173], [-0.19516714086823977, -0.2602524231991969, 0.3253022235640839], [-0.19056515082009318, -0.2710999692645514, 0.3313763269189964], [-0.18399087923310697, -0.28457722307642164, 0.33887584678589766], [-0.17577303960080853, -0.29904061693151734, 0.34687382724167865], [-0.16689777261209882, -0.31580500464498895, 0.3571941593331298], [-0.15736507822355128, -0.3322406782321631, 0.3676243138265914], [-0.14816109722228138, -0.3463753570113456, 0.37673279479605626], [-0.1396145432481224, -0.36018132188100965, 0.3862936775541807], [-0.13073927546822722, -0.3713575788323425, 0.39369938977115077], [-0.12449371654302638, -0.38056155492820515, 0.40040702110236365], [-0.11824815752087511, -0.3874645368718301, 0.40510664532982354], [-0.11331745296110843, -0.39272395161238255, 0.4087455777322099], [-0.11003031655426035, -0.3973259394582111, 0.41227972631137316], [-0.10707189376504267, -0.40225664066766237, 0.41626289216751644], [-0.10444218460072047, -0.40817348204546794, 0.42132382008295344], [-0.10246990271613649, -0.41573389035614056, 0.42817607190653], [-0.10049762082182453, -0.42460915211962486, 0.43634012404842387], [-0.09885405256912966, -0.4361141208055213, 0.44717742572195335], [-0.09753919796210497, -0.44926265607900545, 0.4597290824890823], [-0.09589562969723567, -0.46306861769589186, 0.4728937687153568], [-0.09523820238939307, -0.47818943230826244, 0.48758122232676404], [-0.09359463411504779, -0.4916666796834451, 0.500495833595119], [-0.09425206142559839, -0.5054726399894023, 0.5141848314184605], [-0.09458077508046742, -0.5173063199148471, 0.5258814996162767], [-0.09688177065696921, -0.5274964329357907, 0.5363194609983986], [-0.09852533891777929, -0.535714265850437, 0.544699015094149], [-0.10115504812100973, -0.5422885320752335, 0.551642271567975], [-0.10345604365964414, -0.548534084900955, 0.5582049760328497], [-0.1060857528304466, -0.5560944908388858, 0.5661230163974631], [-0.1087154619839723, -0.5633261833583318, 0.5737206990613581], [-0.11003031655426035, -0.5731875820648644, 0.5836528718291347], [-0.1106877438377864, -0.585021260233898, 0.5954004127992839], [-0.11200259840160343, -0.6001420707867922, 0.6105039616390461], [-0.11101645747914501, -0.6162490206167963, 0.6261689143053809], [-0.10970160291209288, -0.6346569625992535, 0.6440682431677507], [-0.10707189376504267, -0.6524074773988899, 0.6611353167093826], [-0.10444218460072047, -0.6698292783128177, 0.677922880576575], [-0.10016890717182642, -0.6842926597180914, 0.6915853194711825], [-0.09655305700399536, -0.6971124746881563, 0.7037672166154532], [-0.09227977949069568, -0.7050015914223215, 0.7110153314879064], [-0.08899264291084263, -0.7096035761241, 0.7151621674420202], [-0.08439065165347506, -0.7096035761241, 0.7146040983192089], [-0.08044608767622402, -0.7073025837787141, 0.7118627101081048], [-0.07650152365982202, -0.702700599054914, 0.7068526119598125], [-0.07288567327702397, -0.6964550482877871, 0.700258492026044], [-0.06992725021203366, -0.6911956370523529, 0.6947238508950332], [-0.06696882712495675, -0.686922365380997, 0.690179078114598], [-0.06401040401577515, -0.68396394650921, 0.6869526999340757], [-0.06105198088447078, -0.681334240830006, 0.68406409940686], [-0.05940841246862469, -0.6803481011965664, 0.6829369650808306], [-0.05875098510037216, -0.6803481011965664, 0.6828800898049653], [-0.05907969878463515, -0.6803481011965664, 0.682908448922882], [-0.06006583983578334, -0.6790332483488073, 0.6816847199976768], [-0.06269554929348325, -0.6760748294280814, 0.6789756305548977], [-0.06664011344725074, -0.6714728444037357, 0.6747715802343085], [-0.07255695960422626, -0.663583727115445, 0.6675386695012018], [-0.07978866034287696, -0.6537223303204269, 0.6585735459907879], [-0.08734907461074631, -0.6432035068455573, 0.6491075504519852], [-0.09556691604344972, -0.6303836904177982, 0.6375865687001399], [-0.10345604365964414, -0.6159203073605253, 0.624548619395472], [-0.1116738847610535, -0.6021143503877731, 0.6123828438815991], [-0.11759073024973879, -0.5886371062806011, 0.6002676259228599], [-0.12186400749289447, -0.5771321414882868, 0.5898579024316655], [-0.12515114380287323, -0.5656271764087875, 0.5793072686298222], [-0.12613728469062985, -0.5560944908388858, 0.57022074438807], [-0.12482243017308409, -0.5498489381165337, 0.5638390673075023], [-0.12285014838870895, -0.5442608119241725, 0.5579533944295771], [-0.1195630120599196, -0.5399875389073514, 0.5530658695201313], [-0.1149610211544283, -0.5367004057902094, 0.5488746322797623], [-0.1106877438377864, -0.5327558460182888, 0.5441328588704804], [-0.10641446647558184, -0.5301261394846553, 0.5407011766587778], [-0.10378475730693973, -0.5255241530141397, 0.5356742585289023], [-0.10246990271613649, -0.5202647398477764, 0.5302598235690962], [-0.10312733001207844, -0.5143478999625632, 0.5245846055607418], [-0.10575703918504134, -0.5067874933297802, 0.5177046597556066], [-0.10970160291209288, -0.4979122332077099, 0.5098539336509736], [-0.1156184484298711, -0.48969439960509303, 0.5031582560407046], [-0.12252143475703947, -0.480819139145053, 0.4961839845693463], [-0.13073927546822722, -0.47325873194754303, 0.4909853210784956], [-0.1386284023933257, -0.4666844647151091, 0.48683901195010426], [-0.14553138832638368, -0.46241119096196653, 0.4847715900453212], [-0.1511195197097585, -0.4607676241228989, 0.48491639761629957], [-0.15605022380758304, -0.4604389107543559, 0.4861642344795167], [-0.15802250542993873, -0.46306861769589186, 0.4892889298943305], [-0.15966607344125233, -0.4676706048061598, 0.49417512038538186], [-0.15802250542993873, -0.47424487202404514, 0.49987929629407335], [-0.15637893741197428, -0.48312013261455505, 0.5077986161891379], [-0.15276308774902642, -0.4919953930289939, 0.5151660195901617], [-0.15046209249218567, -0.49988451324996525, 0.5220377073203446], [-0.14750366999990816, -0.5071162066642754, 0.5281327292688892], [-0.14618881555195945, -0.5120469066529498, 0.5325065299180279], [-0.14586010193930504, -0.5153340399488096, 0.5355785115813607], [-0.14750366999990816, -0.516320179932904, 0.5369765924780969], [-0.1514482333181451, -0.5156627532770801, 0.5374426876351432], [-0.1567076510160994, -0.5120469066529498, 0.5354897968214132], [-0.16459677743531914, -0.5081023466663224, 0.5340974572397023], [-0.17281461729270303, -0.503171646634506, 0.532021238229174], [-0.18201859773642226, -0.4979122332077099, 0.5301390024322135], [-0.19089386439667327, -0.4942963864410928, 0.5298767640810622], [-0.1997691308647927, -0.4916666796834451, 0.5307012620650322], [-0.20667211576303285, -0.4919953930289939, 0.5336411061712943], [-0.21193153275068627, -0.4946250997847155, 0.5381161249313153], [-0.21488995477676326, -0.5008706532678491, 0.5450221132843338], [-0.21521866833390724, -0.5090884866662126, 0.5527116449429259], [-0.2132463869871169, -0.5209221664969119, 0.562880027280144], [-0.2093018242652489, -0.5340706992793982, 0.5736190072422169], [-0.20305626654506598, -0.5488627982052046, 0.5852198036950458], [-0.1958245680137617, -0.5636548966519603, 0.5967026931039514], [-0.1879354421979616, -0.5781182813388661, 0.6078984106348262], [-0.18004631623022538, -0.5906093859305248, 0.6174432141803049], [-0.17314333088355183, -0.6021143503877731, 0.6265144084315548], [-0.1662403454200604, -0.6083599024023401, 0.6306644300231032], [-0.1603235006439162, -0.6136193145601432, 0.6342178553620039], [-0.15605022380758304, -0.6159203073605253, 0.6353813794639254], [-0.15309180135608064, -0.6142767410756962, 0.6330663585036149], [-0.1524343741417058, -0.6109896084886619, 0.6297178257768331], [-0.1511195197097585, -0.6057301963011648, 0.6242965480830049], [-0.15046209249218567, -0.6011282105883295, 0.619672467390842], [-0.1498046652735464, -0.5955400850185826, 0.6140923632497475], [-0.1491472380538405, -0.5912668124786318, 0.6097879485179504], [-0.14783238361122814, -0.5886371062806011, 0.6069168448268485], [-0.14553138832638368, -0.5869935398992416, 0.6047650790775269], [-0.1429016794133996, -0.5869935398992416, 0.604137654729957], [-0.1392858296301243, -0.5866648266222687, 0.6029727698092914], [-0.13468383895005748, -0.586336113345062, 0.601605995886775], [-0.13041056184299937, -0.5860074000676216, 0.6003428916662713], [-0.12515114380287323, -0.5837064071189924, 0.5969723431675292], [-0.12153529386041878, -0.5794331344696906, 0.5920418777207478], [-0.117262016613767, -0.5735162953514401, 0.5853813471353249], [-0.11430359387790834, -0.5662846029925139, 0.5777054294013472], [-0.11233131204188385, -0.5564232041377004, 0.5676487521063673], [-0.1106877438377864, -0.5452469518454433, 0.556368596465191], [-0.11003031655426035, -0.5343994125940812, 0.545609203314909], [-0.1106877438377864, -0.5225657331155742, 0.5341598281998722], [-0.11200259840160343, -0.5136904733038699, 0.5257589603723979], [-0.11331745296110843, -0.5058013533248564, 0.5183395163122808], [-0.11463230751630296, -0.502185506621665, 0.5151027557559468], [-0.11693330297752613, -0.5028429332971325, 0.5162600245148741], [-0.11824815752087511, -0.5087597733331555, 0.5223209106661205], [-0.1195630120599196, -0.5186211732207597, 0.5322247975862434], [-0.12022043932782811, -0.5337419859644774, 0.5471137556427186], [-0.11923429842556194, -0.5541222110410402, 0.5668052952205431], [-0.11759073024973879, -0.5781182813388661, 0.5899562077467032], [-0.1152897347922843, -0.6050727697735487, 0.615958423653666], [-0.11200259840160343, -0.6323559698909977, 0.6421982985850206], [-0.10772932105342398, -0.6599678816477914, 0.6687026330300374], [-0.10279861636424256, -0.6865936521739255, 0.6942466411383869], [-0.09852533891777929, -0.7089461497408267, 0.7157596563380797], [-0.09392334777045852, -0.7280115144919712, 0.7340452033010665], [-0.08997878388764544, -0.7411600414690598, 0.7466018943321253], [-0.08702036094991306, -0.7503640101415157, 0.755393070484175], [-0.08636293362743236, -0.7533224286064912, 0.7582567096612587], [-0.08570550630386592, -0.7526650022824899, 0.7575289033902948], [-0.0876777882713082, -0.7470768784927337, 0.7522042654323327], [-0.09030749754603731, -0.738530336102118, 0.7440312503222798], [-0.09392334777045852, -0.7283402276707416, 0.7343712157348476], [-0.09819662526615838, -0.7184788322104989, 0.725158196222193], [-0.10214118906776018, -0.7082887233566553, 0.7156156357559388], [-0.1060857528304466, -0.6980986142870198, 0.7061132077953647], [-0.1087154619839723, -0.6898807842344648, 0.6983942641018386], [-0.11200259840160343, -0.6816629540406993, 0.6908031303925912], [-0.1136461666003111, -0.6741025501373847, 0.6836151689983707], [-0.1152897347922843, -0.6668708593348343, 0.6767632274129968], [-0.11660458934101617, -0.6589817419700044, 0.6692186238481476], [-0.11824815752087511, -0.6504351980097214, 0.6610964933858197], [-0.1198917256940083, -0.6409025141791371, 0.6520199832605028], [-0.12186400749289447, -0.6307124036639074, 0.642377593365251], [-0.12515114380287323, -0.6185500134042146, 0.6310839309295725], [-0.12679471194779196, -0.606387622827852, 0.6195020969268279], [-0.13271155721396527, -0.5912668124786318, 0.6059775581296696], [-0.1382996887745252, -0.5784469946219237, 0.5947501403970128], [-0.1442165338720282, -0.5639836099453535, 0.5821305016309096], [-0.1491472380538405, -0.5511637913283285, 0.5709872358385135], [-0.154735369387356, -0.5393301122858216, 0.5610882324177531], [-0.1586799326352621, -0.5288112862121277, 0.5521056940898691], [-0.1613096414459182, -0.5202647398477764, 0.5446982650534928], [-0.16196706864592386, -0.5130330466442197, 0.5379927864523868], [-0.1603235006439162, -0.5077736333325464, 0.5324825701996782], [-0.1567076510160994, -0.5038290733085331, 0.5276372077459273], [-0.1507908061011054, -0.5015280799452373, 0.5237062938118822], [-0.1442165338720282, -0.498898373229919, 0.5193245569521254], [-0.13566997981448808, -0.49659737984139835, 0.5147963685654802], [-0.12679471194779196, -0.49528252647123877, 0.5112550048710104], [-0.1195630120599196, -0.492652819719369, 0.506953759854176], [-0.11298873932163633, -0.4880508328665049, 0.5009591507051067], [-0.1067431801204472, -0.4834488459663749, 0.49509281268106275], [-0.10345604365964414, -0.47687457888406243, 0.48796774171614876], [-0.10148376177019686, -0.46832803153231345, 0.4791973487217575], [-0.10148376177019686, -0.45912405727775113, 0.4702061823011409], [-0.10345604365964414, -0.44794780256925676, 0.45973947709146323], [-0.10509961189342096, -0.43578540741866695, 0.4482798788025191], [-0.1067431801204472, -0.4239517253284841, 0.43718322464525633], [-0.10740060740936822, -0.41047447589297886, 0.42429257103031737], [-0.10740060740936822, -0.3986407931195172, 0.4128551470078325], [-0.10509961189342096, -0.3871358234484324, 0.4011484441166929], [-0.10049762082182453, -0.3769457071995947, 0.3901125965244519], [-0.09392334777045852, -0.36839915790279604, 0.38018355408920534], [-0.08504807897921357, -0.3637971697498838, 0.37360615152333926], [-0.07485795530808936, -0.362153602540519, 0.36980933642349284], [-0.06269554929348325, -0.3628110294250167, 0.368188233073318], [-0.05020442921345694, -0.36708430414982757, 0.37050151290623917], [-0.03672716763043671, -0.3743159997416429, 0.3761134835455116], [-0.023578619298789433, -0.38450611605229307, 0.38522837975629043], [-0.010430070525272339, -0.39633979920962775, 0.3964770142248983], [0.003047192427820339, -0.4098170490806396, 0.40982837761538127], [0.014880887113591354, -0.42362301193254476, 0.4238842967604349], [0.027372009674298106, -0.4361141208055213, 0.43697225687631785], [0.038548277571306064, -0.44827651594706014, 0.44993088852994895], [0.048738404466217605, -0.45780920379725293, 0.46039624146096947], [0.056627535151335326, -0.4647121845264523, 0.46814964721193925], [0.06155824191206011, -0.4676706048061598, 0.47170458101131796], [0.06780380390026441, -0.46931417161972416, 0.47418682763912096], [0.06878994527615954, -0.4666844647151091, 0.4717270886619984], [0.06813251769194636, -0.4604389107543559, 0.4654525008029295], [0.06451666599900902, -0.45287850321068285, 0.45745091415579897], [0.05892853163176645, -0.4433458152543596, 0.44724499297793024], [0.05169682845410899, -0.4334844137038221, 0.4365561808019215], [0.042164129019213736, -0.4249378655148263, 0.4270245933482585], [0.03164528853782095, -0.4183635975640411, 0.4195587253929644], [0.021126448343487966, -0.4154051769540436, 0.41594204867965723], [0.010607608435402774, -0.4170487439620629, 0.4171836240758416], [0.0004174825466486398, -0.4242804387241775, 0.42428064412091354], [-0.009115215623556744, -0.4361141208055213, 0.4362093689065341], [-0.016346917528137828, -0.45287850321068285, 0.4531734330066362], [-0.022921191870621138, -0.4749022987405021, 0.4754551234194274], [-0.02752318384460778, -0.5002132265895001, 0.5009698570812645], [-0.030810320935775404, -0.5278251462552324, 0.5287236148457177], [-0.034097457999380715, -0.5570806307346219, 0.558123163631204], [-0.03705588133308016, -0.5837064071189924, 0.5848814478619869], [-0.03837073614090267, -0.6100034687080311, 0.611209084706555], [-0.04100044574334666, -0.6313698301554347, 0.6326996909922239], [-0.04428758272166619, -0.6484629186123119, 0.6499734969970131], [-0.047574719672524995, -0.6616114477728732, 0.6633197281673723], [-0.051519283977342234, -0.6685144254359896, 0.6704966619138005], [-0.05710741667495384, -0.671801557621237, 0.674224435823567], [-0.06335297665517553, -0.6695005650939518, 0.6724913429273213], [-0.0695985365367828, -0.665556006449812, 0.6691851418026884], [-0.07650152365982202, -0.6589817419700044, 0.6634074308990635], [-0.08307579699873885, -0.6517500509367491, 0.6570233762531061], [-0.08932135657004811, -0.6448470730289735, 0.651003880428948], [-0.09490948873506563, -0.6389302347418218, 0.645940907451441], [-0.09852533891777929, -0.6349856758423693, 0.6425838863011224], [-0.10148376177019686, -0.6330133963802218, 0.6410966494217966], [-0.10312733001207844, -0.633670822868525, 0.642007755366159], [-0.10312733001207844, -0.6353143890852553, 0.6436300328404442], [-0.10214118906776018, -0.6386015215014651, 0.6467184285051433], [-0.09984019352155787, -0.6425460803705849, 0.65025651064947], [-0.09753919796210497, -0.6461619259715781, 0.6534823101770926], [-0.09556691604344972, -0.6487916318457858, 0.6557923581402679], [-0.09523820238939307, -0.6497777715448341, 0.6567202354032755], [-0.09556691604344972, -0.6497777715448341, 0.6567679863055342], [-0.09655305700399536, -0.6471480656761246, 0.6543111734680728], [-0.10016890717182642, -0.6418886538946944, 0.6496574897303508], [-0.10641446647558184, -0.6346569625992535, 0.6435165101619329], [-0.11200259840160343, -0.627425271192444, 0.6373437478940408], [-0.11923429842556194, -0.6178925868946805, 0.6292917184108149], [-0.12679471194779196, -0.6093460421864507, 0.6223981829232917], [-0.1343551253280451, -0.6001420707867922, 0.6149974022954681]] caption="Signals vs time"
  in  "Update\nmodulation":bool=TRUE
  out "Present modulation":dbl=0.27257525083612044
  in  "N voltages":dbl=30.0
  in  "Ending V":dbl=0.4
  in  "Starting V":dbl=0.1
  out "PSHet Optimization Errors":errorcluster
  in  "time":dbl=1.0 caption="recording time [s]"
  # "Input / Output settings"
  # "Amplitude / Phase"
  # "Should be sidebands:\n+1,+2,-1,-2\n(Im,Re,Im,Re)\n(Negative sidebands can be supplied as zero)"
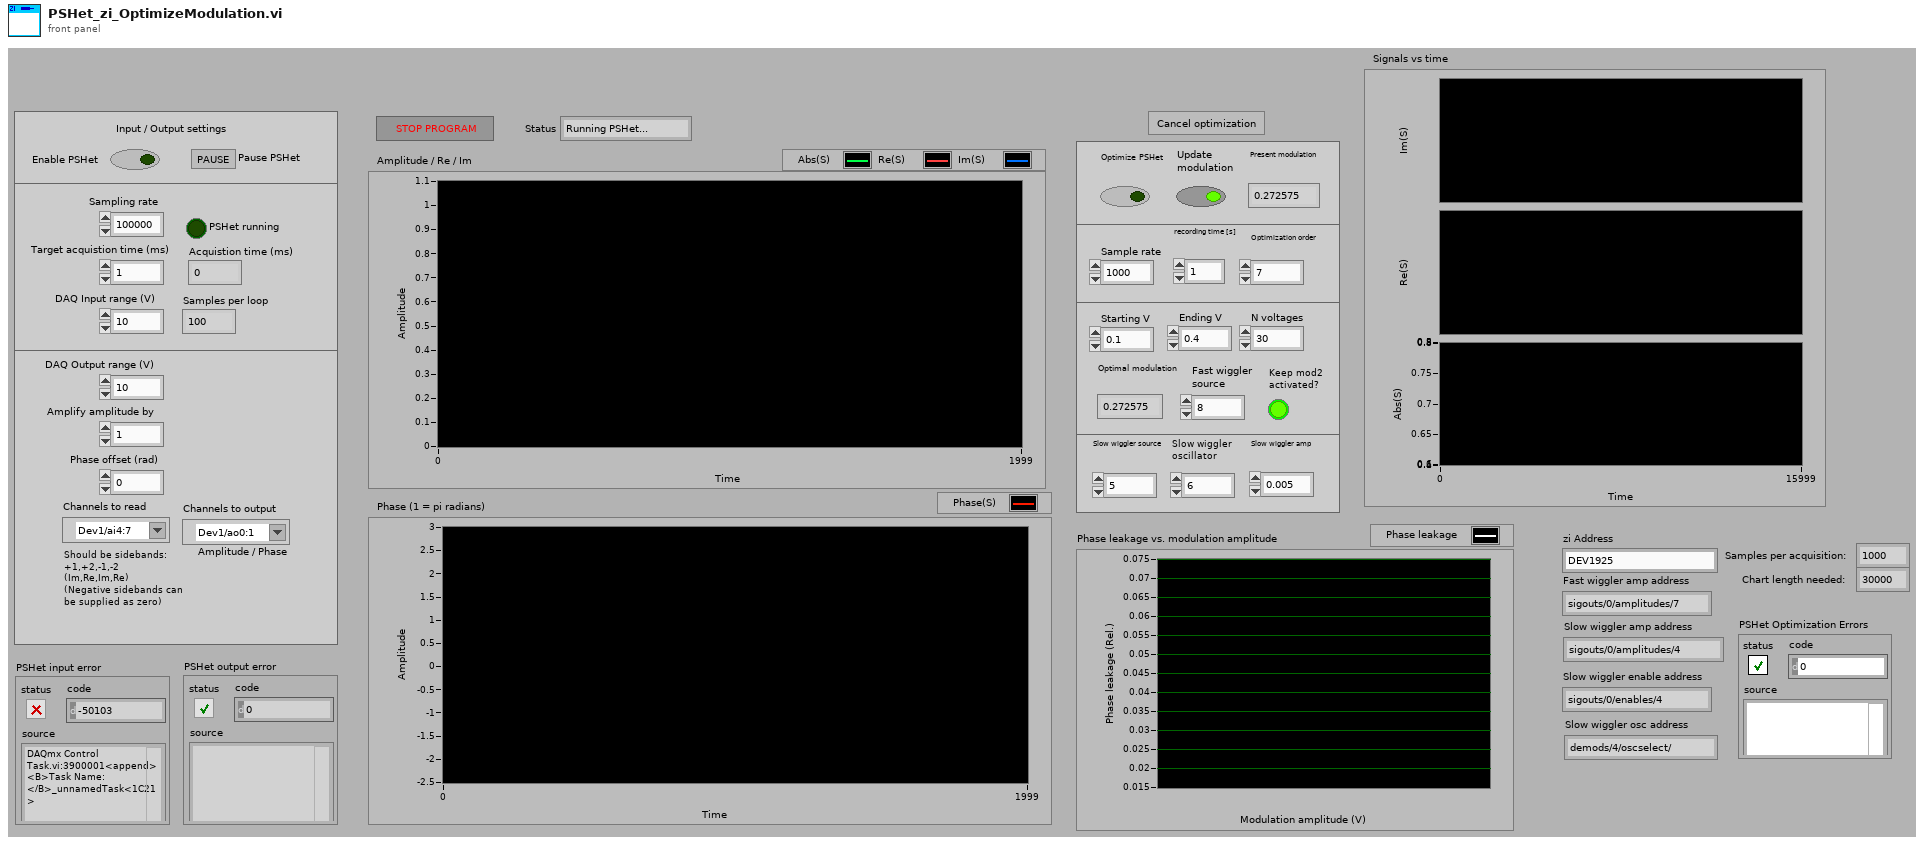
[diagram p1: front panel]
types:
  T1 = cluster{"[0]":dbl, "[1]":dbl, "[2]":dbl, "[3]":dbl, "[4]":dbl, "[5]":dbl, "[6]":dbl, "[7]":dbl, "[8]":dbl}
  T2 = typedef "zi_OptimizeModulation_Control.ctl" = enum16{"Sit Idle", "Disable PSHet", "Prepare optimization", "Enable wiggling", "Measure phase leakages", "Fit phase leakages", "Set optimal amplitude"}
  T3 = typedef "PSHet_DAQInAndOut_control.ctl" = enum16{"Prepare DAQ task", "Run DAQ task", "Pause", "Close DAQ task", "Sit Idle"}
  T4 = typedef "Zurich Instruments LabOne.lvlib/ziTypeHandle.ctl" = cluster{"handleValid":bool, "Conn":u64, "Path Prefix":string, "Handle":u64, "Connected":bool, "Clockbase(s)":dbl}
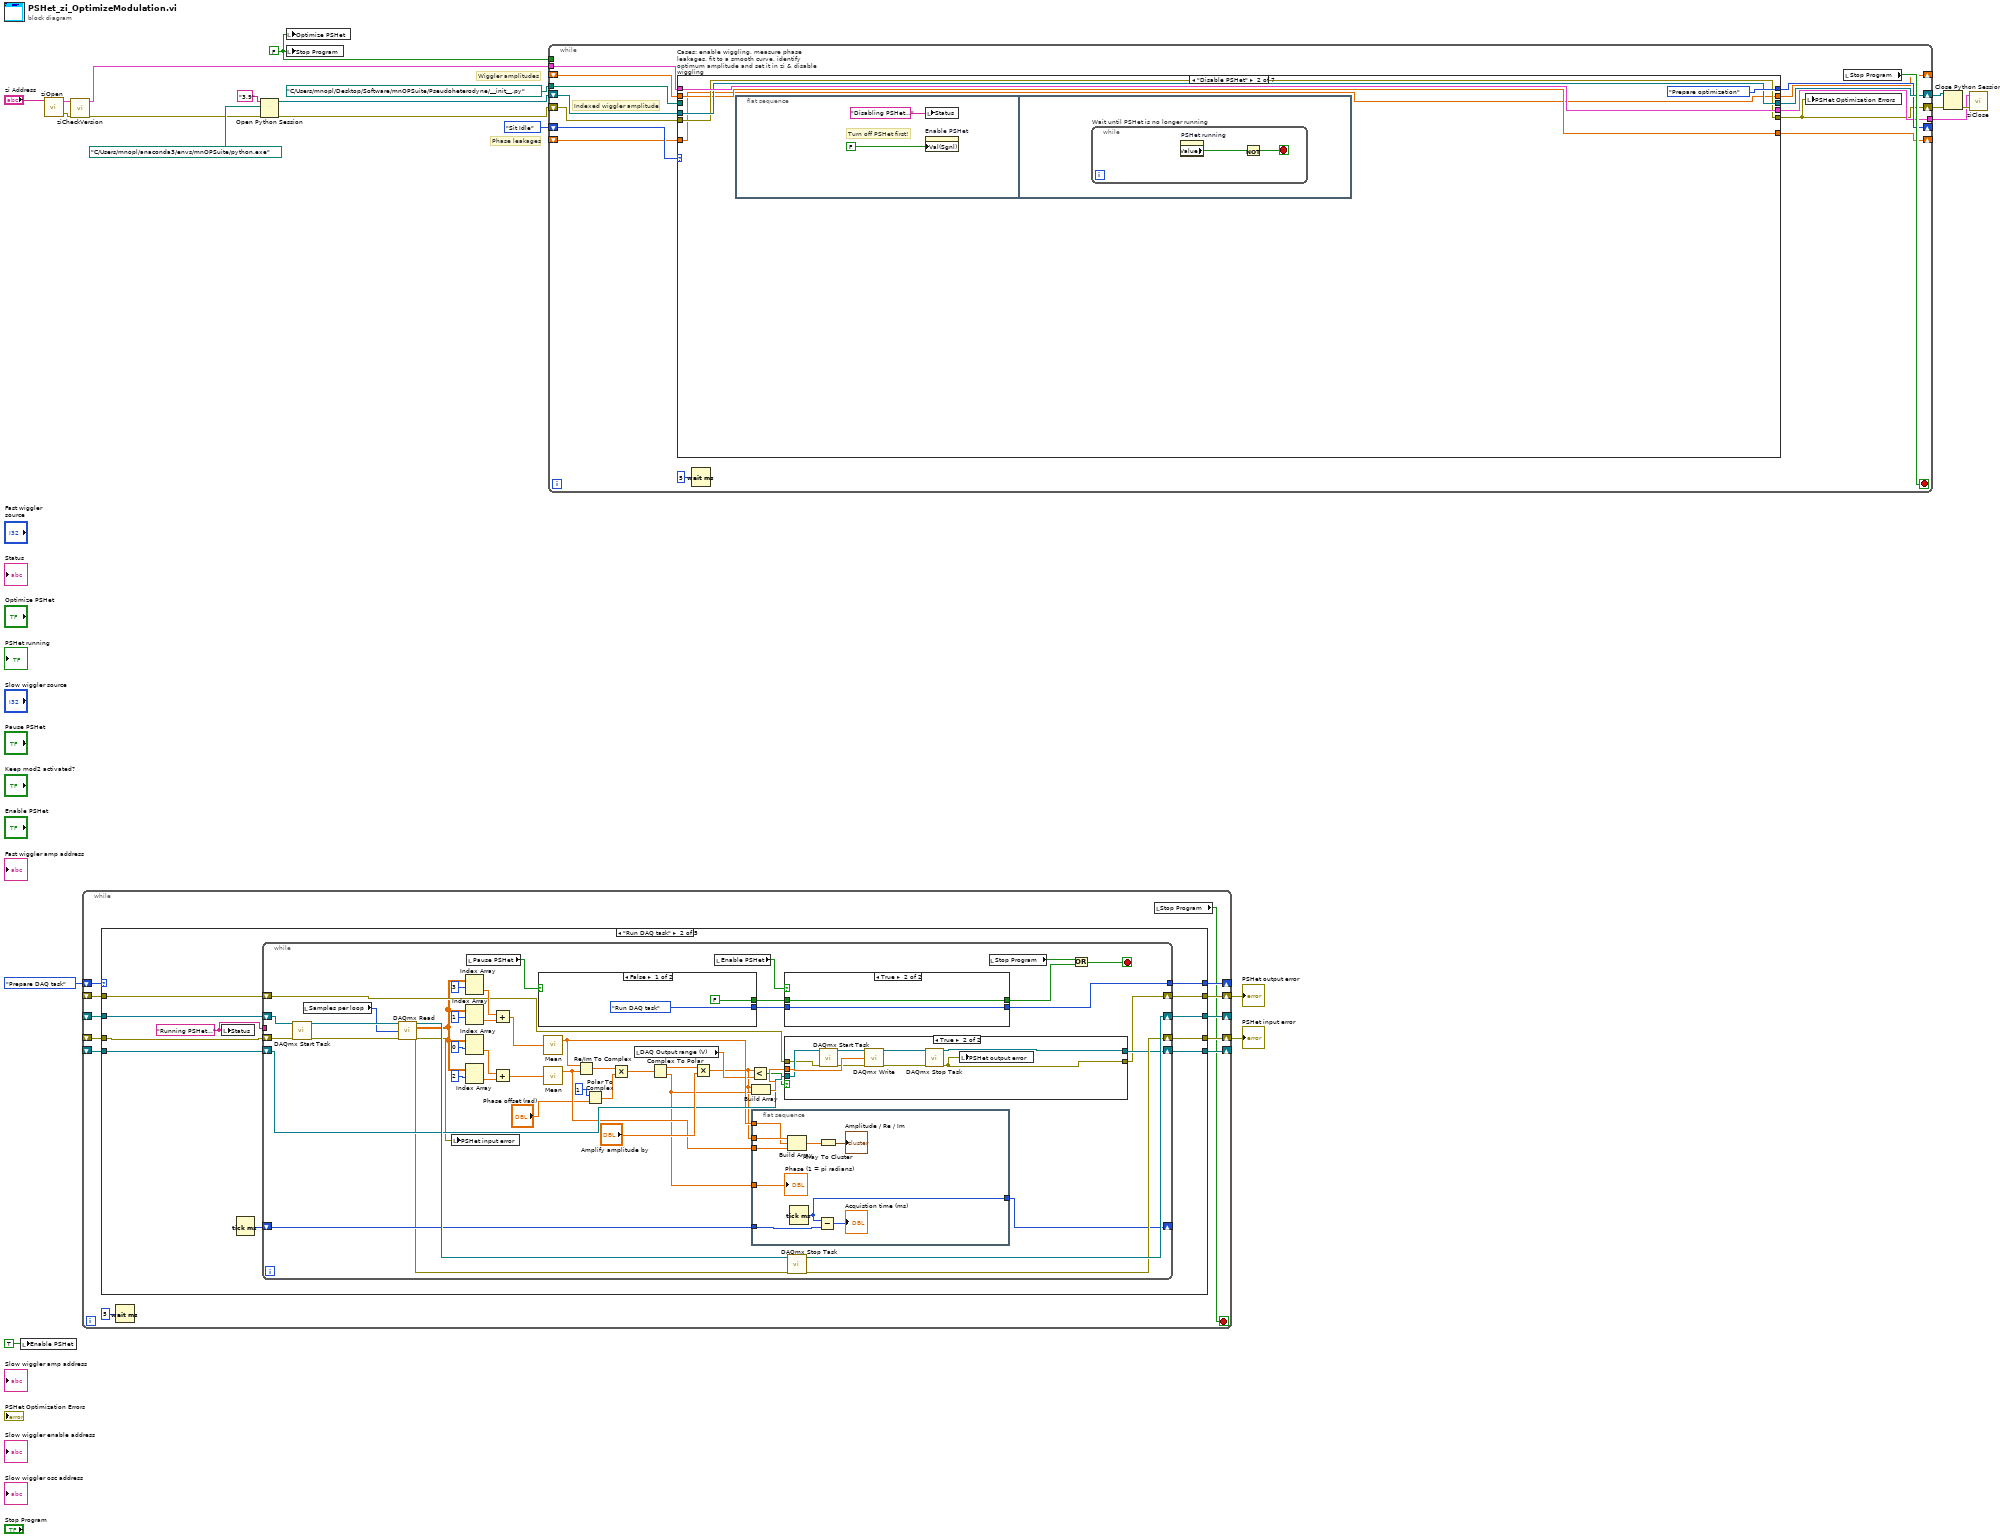
[diagram p0: block diagram]
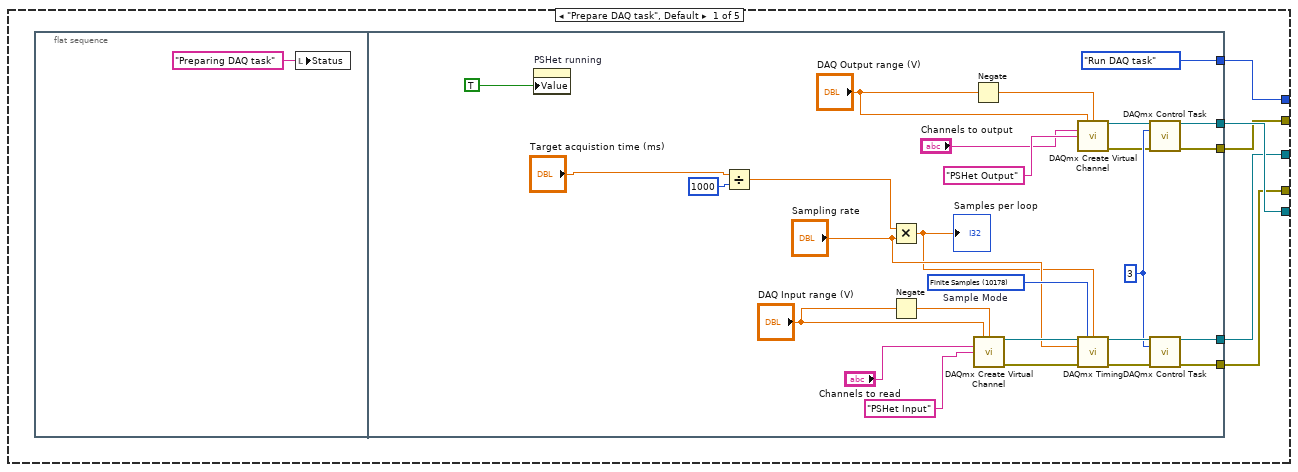
[diagram p2: hidden frame]
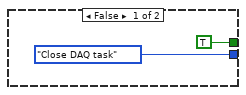
[diagram p4: hidden frame]
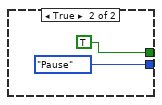
[diagram p5: hidden frame]
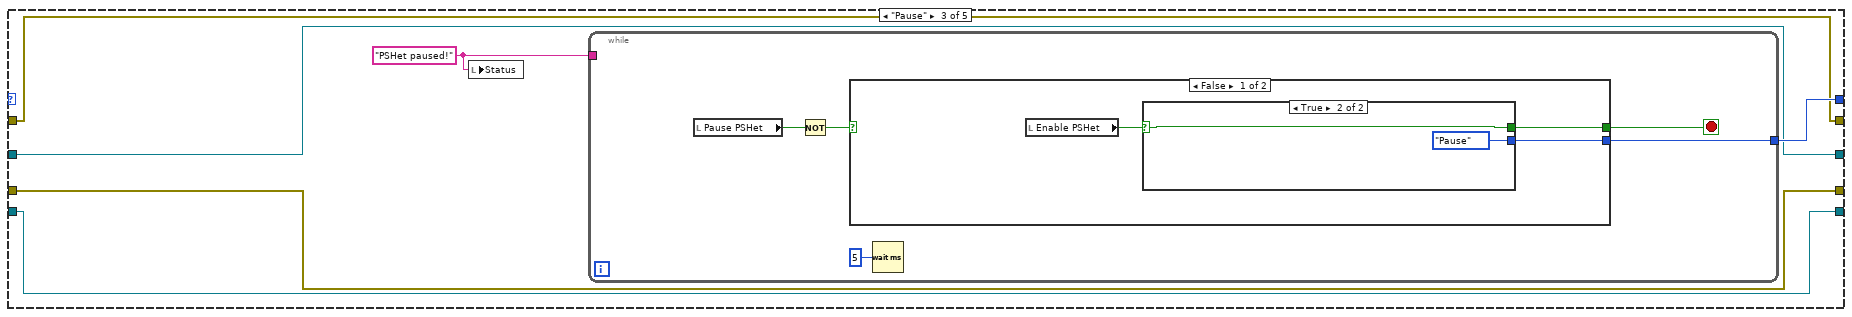
[diagram p6: hidden frame]
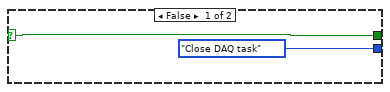
[diagram p7: hidden frame]
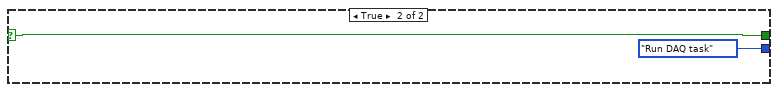
[diagram p8: hidden frame]
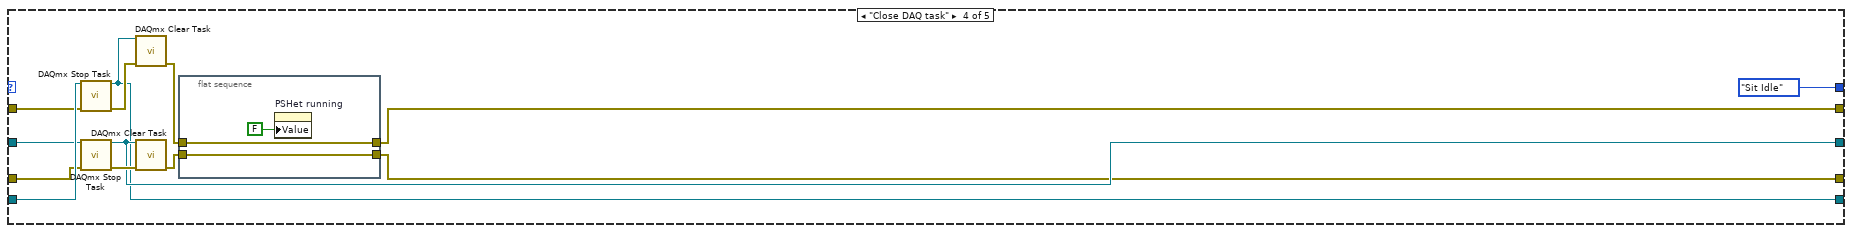
[diagram p9: hidden frame]
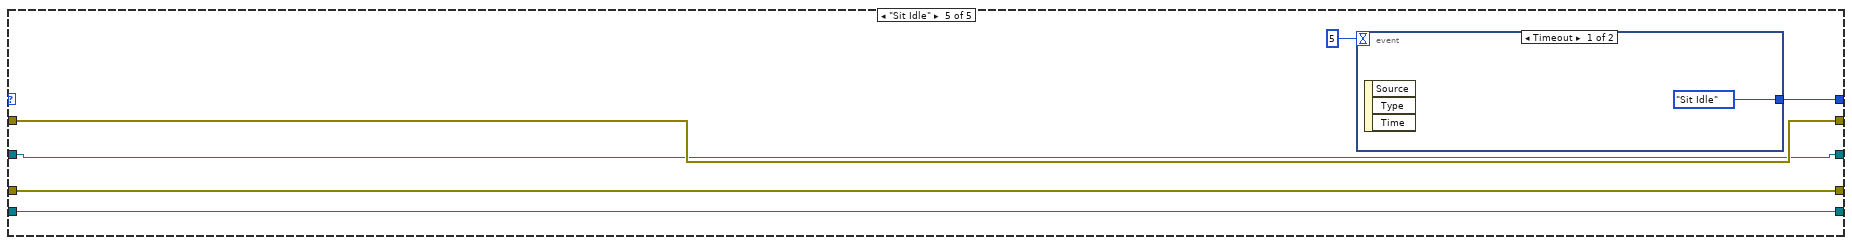
[diagram p10: hidden frame]
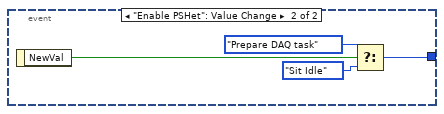
[diagram p11: hidden frame]
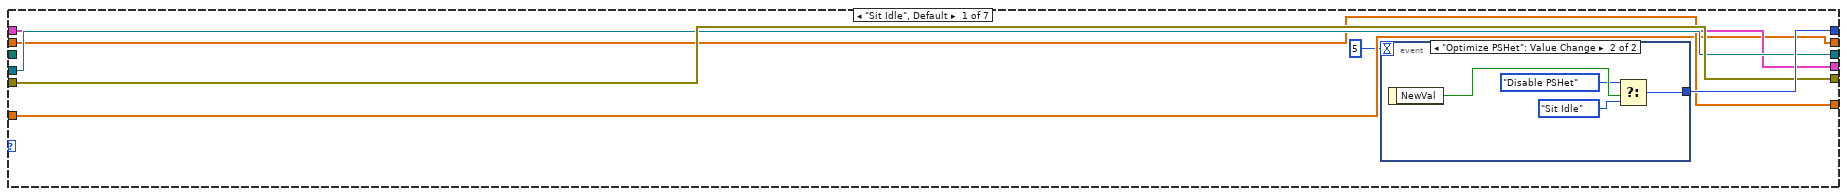
[diagram p12: hidden frame]
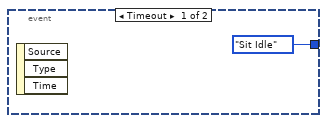
[diagram p13: hidden frame]
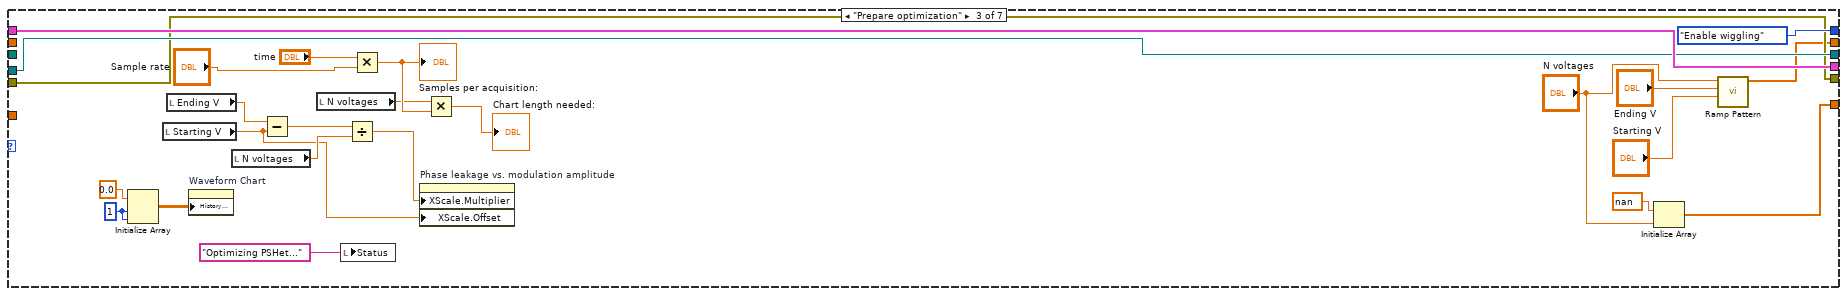
[diagram p14: hidden frame]
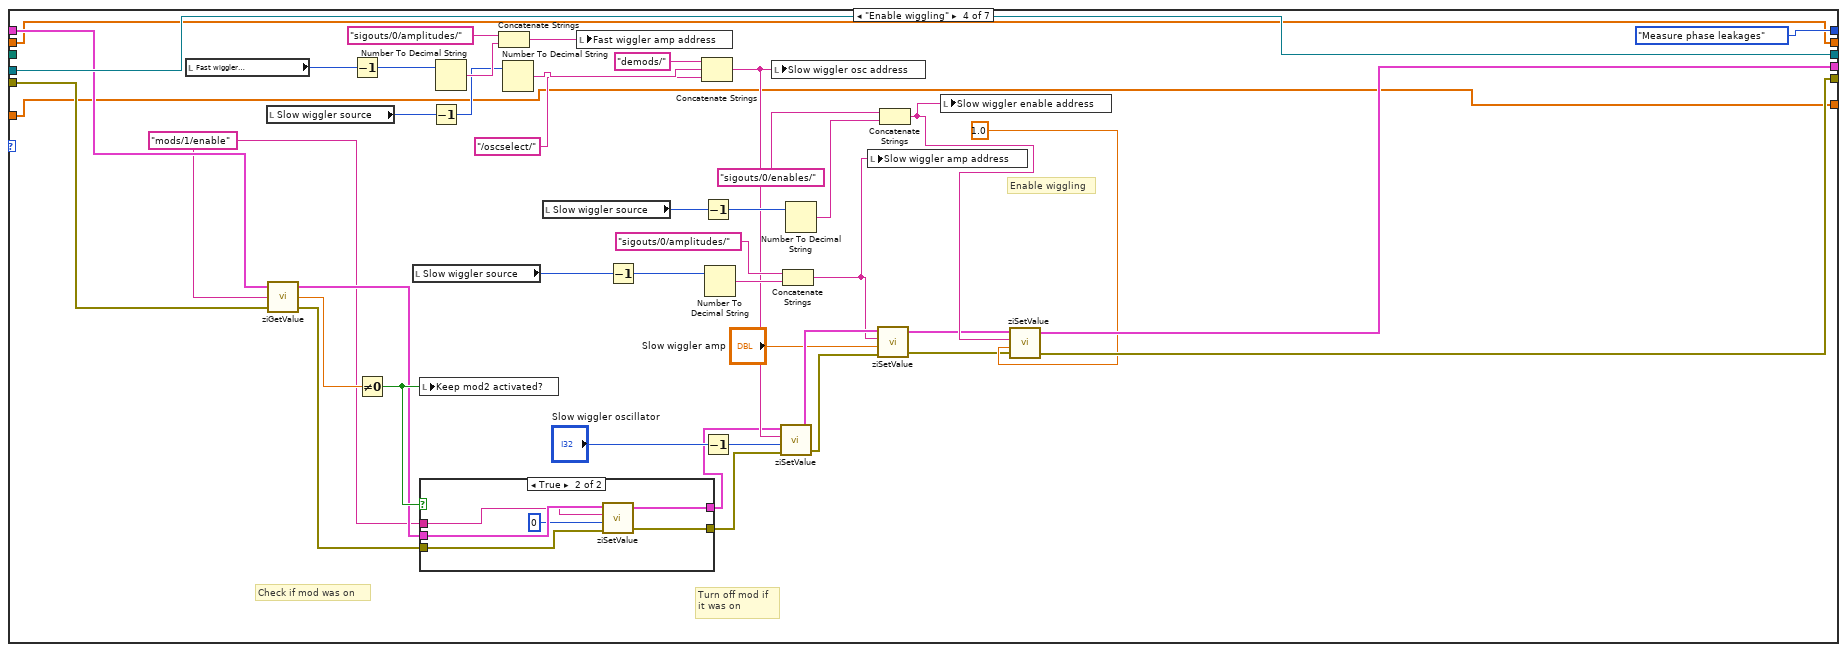
[diagram p15: hidden frame]
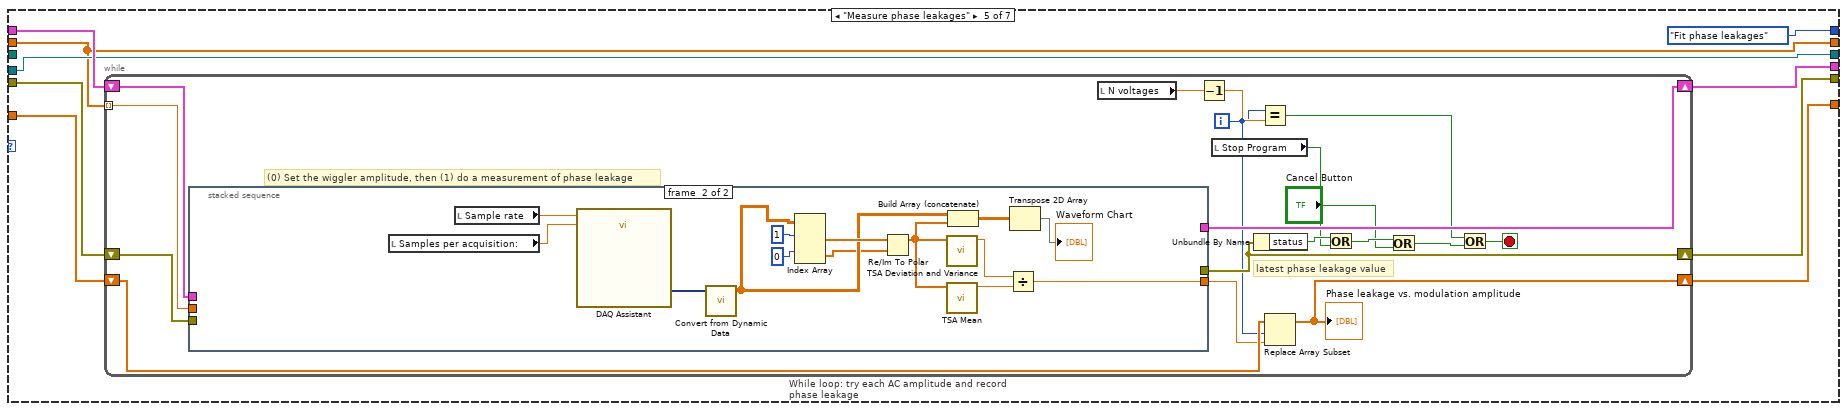
[diagram p17: hidden frame]
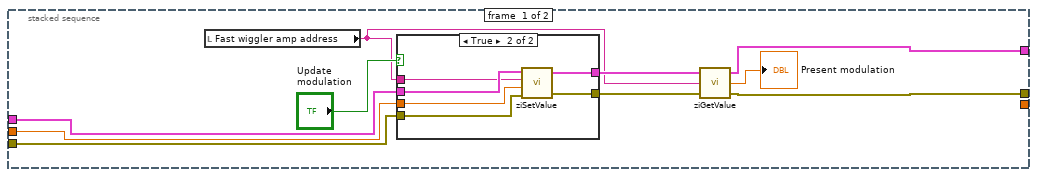
[diagram p18: hidden frame]
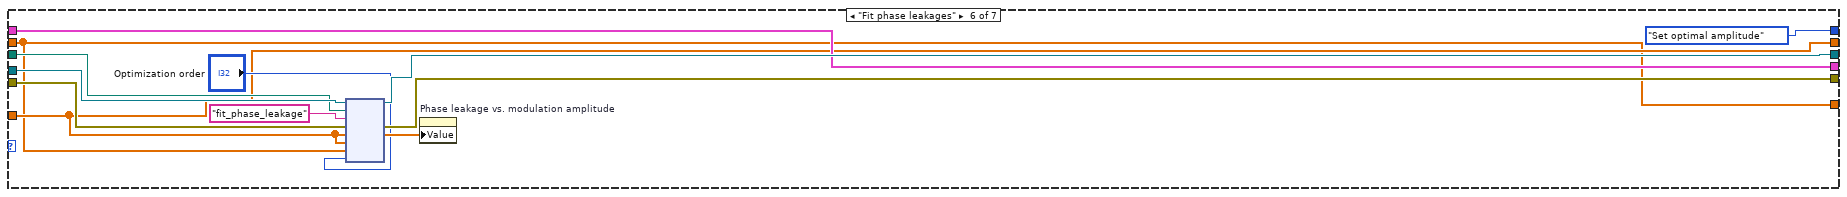
[diagram p20: hidden frame]
diagram:
  w6 = FALSE
  # "Phase leakages"
  # "Wiggler amplitudes"
  n1 = local write "Enable PSHet"(TRUE) -> ()
  n2 = call <instrlib>:"ziOpen.vi"("Address"="zi Address") -> ("Error Out"=w18:errorcluster, "HandleOut"=w19:T4)  [unwired: 1 in, 3 out]
  n3 = call <instrlib>:"ziCheckVersion.vi"("Handle In"=w19, "Error In"=w18) -> ("Handle Out"=w17:T4, "Error Out"=w15:errorcluster)  [unwired: 11 in, 1 out]
  n4 = while {
    shift-right: [w31] -> _
    shift-left: _ -> [w24]
    shift-right: [w30] -> w3
    shift-left: _ -> [w23]
    shift-right: [w29] -> _
    shift-left: _ -> [w26]
    shift-right: [w28] -> w4
    shift-left: _ -> [w25]
    shift-right: [w27] -> _
    shift-left: PSHet_DAQInAndOut_control."Prepare DAQ task" -> [w32]
    stop <- w22 stop-if-true
    n5 = case shown="\"Run DAQ task\"" w32 {
      tunnel: [w36 w69 w156 w177 w192] -> w29
      tunnel: [w35 w70 w155 w175 w191] -> w28
      tunnel: [w34 w72 w154 w179 w190] -> w31
      tunnel: [w33 w71 w153 w173 w193] -> w30
      tunnel: [w37 w68 w157 PSHet_DAQInAndOut_control."Sit Idle" w194] -> w27
      tunnel: w26 -> [_ w76 w156 w185 w192]
      tunnel: w25 -> [_ w75 w155 w184 w191]
      tunnel: w24 -> [_ w74 w154 w183 w190]
      tunnel: w23 -> [_ w73 w153 w182 w193]
      frame "Prepare DAQ task", Default {
        n6 = flat-sequence {
          tunnel: [PSHet_DAQInAndOut_control."Run DAQ task"] -> w37
          tunnel: [w51] -> w36
          tunnel: [w50] -> w35
          tunnel: [w49] -> w34
          tunnel: [w48] -> w33
          frame #0 {
            n7 = local write "Status"("Preparing DAQ task") -> ()
          }
          frame #1 {
            w56 = 3
            w55 = 10178 items=["Finite Samples"=10178, "Continuous Samples"=10123, "Hardware Timed Single Point"=12522]  # Sample Mode
            n8 = property on="PSHet running" class="Bool (strict)"("Value"=TRUE ("PSHet running")) -> ()  [unwired: 2 in, 2 out]
            n9 = Divide(x="Target acquistion time (ms)", y=1000) -> (x/y=w42:dbl)
            n10 = Multiply(x=w42, y="Sampling rate") -> (x*y=w45:dbl)
            "Samples per loop" <- w45
            n11 = Negate(x="DAQ Input range (V)") -> (-x=w59:dbl)
            n12 = Negate(x="DAQ Output range (V)") -> (-x=w65:dbl)
            n13 = call-poly <vilib>:"DAQmx Create Virtual Channel.vi"("maximum value"="DAQ Input range (V)", "minimum value"=w59, "physical channels"="Channels to read", "name to assign"="PSHet Input") -> ("task out"=w58:refnum<k21>, "error out"=w57:errorcluster)  [unwired: 10 in]
            n14 = call-poly <vilib>:"DAQmx Create Virtual Channel.vi"("maximum value"="DAQ Output range (V)", "minimum value"=w65, "physical channels"="Channels to output", "name to assign"="PSHet Output") -> ("task out"=w41:refnum<k21>, "error out"=w40:errorcluster)  [unwired: 10 in]
            n15 = call-poly <vilib>:"DAQmx Timing.vi"("task/channels in"=w58, "sample mode"=w55, "samples per channel"=w45, "rate"="Sampling rate", "error in"=w57) -> ("task out"=w62:refnum<k21>, "error out"=w63:errorcluster)  [unwired: 9 in]
            n16 = call <vilib>:"DAQmx Control Task.vi"("task/channels in"=w41, "action"=w56, "error in"=w40) -> ("task out"=w51:refnum<k21>, "error out"=w50:errorcluster)  [unwired: 11 in]
            n17 = call <vilib>:"DAQmx Control Task.vi"("task/channels in"=w62, "action"=w56, "error in"=w63) -> ("task out"=w49:refnum<k21>, "error out"=w48:errorcluster)  [unwired: 11 in]
          }
        }
      }
      frame "Run DAQ task" {
        w67 = "Running PSHet..."
        n18 = local write "Status"(w67) -> ()
        n19 = Tick Count (ms)() -> (millisecond timer value=w66:u32)
        n20 = while {
          shift-right: [w82] -> w69
          shift-left: w76 -> [w103]
          shift-right: [w81] -> w70
          shift-left: w75 -> [w102]
          shift-right: [w106] -> w72
          shift-left: w74 -> [w110]
          shift-right: [w105] -> w71
          shift-left: w73 -> [w108]
          tunnel: [w90] -> w68
          tunnel: w67 -> [_]
          shift-right: [w84] -> _
          shift-left: w66 -> [w83]
          stop <- w86 stop-if-true
          n21 = call <vilib>:"DAQmx Start Task.vi"("task/channels in"=w110, "error in"=w108) -> ("task out"=w109:refnum<k21>, "error out"=w107:errorcluster)  [unwired: 12 in]
          n22 = local read "Samples per loop"() -> (w101:i32)
          n23 = call-poly <vilib>:"DAQmx Read.vi"("task/channels in"=w109, "number of samples per channel"=w101, "error in"=w107) -> ("task out"=w104:refnum<k21>, "data"=w100:dbl[][], "error out"=w77:errorcluster)  [unwired: 10 in]
          n24 = local write "PSHet input error"(w77) -> ()
          n25 = Index Array(array=w100, index (row)=3) -> (element=w121:dbl[])  [unwired: 1 in]
          n26 = Index Array(array=w100, index (row)=1) -> (element=w122:dbl[])  [unwired: 1 in]
          n27 = Index Array(array=w100, index (row)=0) -> (element=w117:dbl[])  [unwired: 1 in]
          n28 = Index Array(array=w100, index (row)=2) -> (element=w116:dbl[])  [unwired: 1 in]
          n29 = local read "Pause PSHet"() -> (w113:bool)
          n30 = Add(x=w121, y=w122) -> (x+y=w120:dbl[])
          n31 = Add(x=w117, y=w116) -> (x+y=w115:dbl[])
          n32 = case shown="False" w113 {
            tunnel: [PSHet_DAQInAndOut_control."Run DAQ task" PSHet_DAQInAndOut_control."Pause"] -> w89
            tunnel: [FALSE TRUE] -> w88
            frame False {
            }
            frame True {
            }
          }
          n33 = call-poly <vilib>:"Mean.vi"("X"=w120) -> ("mean"=w99:dbl)  [unwired: 1 out]
          n34 = call-poly <vilib>:"Mean.vi"("X"=w115) -> ("mean"=w98:dbl)  [unwired: 1 out]
          n35 = Re/Im To Complex(1:w98, 2:w99) -> (0:w94:cdb)
          n36 = Polar To Complex(1:"Phase offset (rad)", 2:1) -> (0:w92:cdb)
          n37 = Multiply(x=w94, y=w92) -> (x*y=w93:cdb)
          n38 = local read "DAQ Output range (V)"() -> (w80:dbl)
          n39 = Complex To Polar(r * e^(i*theta)=w93) -> (r=w112:dbl, theta=w97:dbl)
          n40 = Multiply(x=w112, y="Amplify amplitude by") -> (x*y=w79:dbl)
          n41 = local read "Enable PSHet"() -> (w91:bool)
          n42 = Less?(x=w79, y=w80) -> (x < y?=w78:bool)
          n43 = Build Array(w79, w97) -> (w114:dbl[])
          n44 = flat-sequence {
            tunnel: w79 -> [w147]
            tunnel: w97 -> [w141]
            tunnel: w99 -> [w145]
            tunnel: w98 -> [w144]
            tunnel: [w140] -> w84
            tunnel: w83 -> [w142]
            frame #0 {
              n45 = Build Array(w147, w145, w144) -> (w148:dbl[])
              n46 = Tick Count (ms)() -> (millisecond timer value=w140:u32)
              n47 = Subtract(x=w140, y=w142) -> (x-y=→"Acquistion time (ms)":u32)
              n48 = Array To Cluster(array=w148) -> (cluster=→"Amplitude / Re / Im":T1)
              "Phase (1 = pi radians)" <- w141
            }
          }
          n49 = case shown="True" w91 {
            tunnel: [PSHet_DAQInAndOut_control."Close DAQ task" w139] -> w90
            tunnel: [TRUE w138] -> w87
            tunnel: w89 -> [_ w139]
            tunnel: w88 -> [_ w138]
            frame False {
            }
            frame True {
            }
          }
          n50 = case shown="True" w78 {
            tunnel: w114 -> [_ w135]
            tunnel: w103 -> [w126 w134]
            tunnel: w102 -> [w125 w133]
            tunnel: [w126 w128] -> w82
            tunnel: [w125 w127] -> w81
            frame False {
            }
            frame True {
              n51 = call <vilib>:"DAQmx Start Task.vi"("task/channels in"=w134, "error in"=w133) -> ("task out"=w132:refnum<k21>, "error out"=w131:errorcluster)  [unwired: 12 in]
              n52 = call-poly <vilib>:"DAQmx Write.vi"("task/channels in"=w132, "data"=w135, "error in"=w131) -> ("task out"=w130:refnum<k21>, "error out"=w129:errorcluster)  [unwired: 10 in, 1 out]
              n53 = call <vilib>:"DAQmx Stop Task.vi"("task/channels in"=w130, "error in"=w129) -> ("task out"=w128:refnum<k21>, "error out"=w127:errorcluster)  [unwired: 12 in]
              n54 = local write "PSHet output error"(w127) -> ()
            }
          }
          n55 = call <vilib>:"DAQmx Stop Task.vi"("task/channels in"=w104, "error in"=w77) -> ("task out"=w106:refnum<k21>, "error out"=w105:errorcluster)  [unwired: 12 in]
          n56 = local read "Stop Program"() -> (w85:bool)
          n57 = Or(x=w85, y=w87) -> (x .or. y?=w86:bool)
        }
      }
      frame "Pause" {
        w158 = "PSHet paused!"
        n58 = local write "Status"(w158) -> ()
        n59 = while {
          tunnel: w158 -> [_]
          tunnel: [w162] -> w157
          stop <- w161 stop-if-true
          n60 = local read "Pause PSHet"() -> (w160:bool)
          n61 = Not(x=w160) -> (.not. x?=w159:bool)
          n62 = case shown="False" w159 {
            selector: w159 -> [_ w172]
            tunnel: [w164 w172] -> w161
            tunnel: [w165 PSHet_DAQInAndOut_control."Run DAQ task"] -> w162
            frame False {
              n63 = local read "Enable PSHet"() -> (w166:bool)
              n64 = case shown="True" w166 {
                selector: w166 -> [w168 w170]
                tunnel: [PSHet_DAQInAndOut_control."Close DAQ task" PSHet_DAQInAndOut_control."Pause"] -> w165
                tunnel: [w168 w170] -> w164
                frame False {
                }
                frame True {
                }
              }
            }
            frame True {
            }
          }
          n65 = Wait (ms)(milliseconds to wait=5) -> ()  [unwired: 1 out]
        }
      }
      frame "Close DAQ task" {
        n66 = call <vilib>:"DAQmx Stop Task.vi"("task/channels in"=w185, "error in"=w184) -> ("task out"=w177:refnum<k21>, "error out"=w178:errorcluster)  [unwired: 12 in]
        n67 = call <vilib>:"DAQmx Stop Task.vi"("task/channels in"=w183, "error in"=w182) -> ("task out"=w179:refnum<k21>, "error out"=w180:errorcluster)  [unwired: 12 in]
        n68 = call <vilib>:"DAQmx Clear Task.vi"("task in"=w177, "error in"=w178) -> ("error out"=w176:errorcluster)  [unwired: 13 in]
        n69 = call <vilib>:"DAQmx Clear Task.vi"("task in"=w179, "error in"=w180) -> ("error out"=w174:errorcluster)  [unwired: 13 in]
        n70 = flat-sequence {
          tunnel: w176 -> [w187]
          tunnel: [w187] -> w175
          tunnel: w174 -> [w186]
          tunnel: [w186] -> w173
          frame #0 {
            n71 = property on="PSHet running" class="Bool (strict)"("Value"=FALSE ("PSHet running")) -> ()  [unwired: 2 in, 2 out]
          }
        }
      }
      frame "Sit Idle" {
        n72 = event shown="[0] Timeout" {
          selector: _ -> [_ _]
          dyn-events: _ -> [_ _]
          timeout: 5 -> [_ _]
          tunnel: [PSHet_DAQInAndOut_control."Sit Idle" w196] -> w194
          event Timeout {
            n73 = event-data() -> ()  [unwired: 1 in, 3 out]
          }
          event "Enable PSHet": Value Change {
            n74 = event-data() -> ("NewVal"=w199:bool)  [unwired: 1 in]
            n75 = Select(t=PSHet_DAQInAndOut_control."Prepare DAQ task", s=w199, f=PSHet_DAQInAndOut_control."Sit Idle") -> (s? t:f=w196:T3)
          }
        }
      }
    }
    n76 = Wait (ms)(milliseconds to wait=5) -> ()  [unwired: 1 out]
    n77 = local read "Stop Program"() -> (w22:bool)
  }
  "PSHet output error" <- w4
  "PSHet input error" <- w3
  n78 = Open Python Session(python version="3.9", python path=path "C:/Users/mnopl/anaconda3/envs/mnOPSuite/python.exe", 3:w15) -> (session out=w14:refnum<k35>, error out=w7:errorcluster)
  n79 = local write "Optimize PSHet"(w6) -> ()
  n80 = local write "Stop Program"(w6) -> ()
  n81 = while {
    tunnel: w17 -> [w214]
    tunnel: path "C:/Users/mnopl/Desktop/Software/mnOPSuite/Pseudoheterodyne/__init__.py" -> [w212]
    tunnel: [w201] -> w9
    shift-right: [w210] -> w8
    shift-left: w14 -> [w213]
    shift-right: [w200] -> w10
    shift-left: w7 -> [w209]
    tunnel: w6 -> [_]
    shift-right: [w203] -> _
    shift-left: _ -> [w206]
    shift-right: [w207] -> _
    shift-left: zi_OptimizeModulation_Control."Sit Idle" -> [w208]
    shift-right: [w202] -> _
    shift-left: _ -> [w205]
    stop <- w211 stop-if-true
    # "Indexed wiggler amplitude"
    n82 = case "Cases: enable wiggling, measure phase leakages, fit to a smooth curve, identify optimum amplitude and set it in zi & disable wiggling" shown="\"Disable PSHet\"" w208 {
      tunnel: w214 -> [w218 w231 w258 w300 w321 w376 w402]
      tunnel: [w220 w229 w256 w302 w320 w377 w387] -> w200
      tunnel: [w218 w231 w258 w304 w319 w376 w388] -> w201
      tunnel: w209 -> [w220 w229 w256 w299 w318 w379 w404]
      tunnel: [w219 w230 w257 w303 w317 w381 w405] -> w210
      tunnel: w213 -> [w219 w230 w257 w303 w317 w380 w406]
      tunnel: w212 -> [_ _ _ _ _ w378 w407]
      tunnel: [w217 w228 w260 w262 w314 w373 w394] -> w202
      tunnel: [w221 zi_OptimizeModulation_Control."Prepare optimization" zi_OptimizeModulation_Control."Enable wiggling" zi_OptimizeModulation_Control."Measure phase leakages" zi_OptimizeModulation_Control."Fit phase leakages" zi_OptimizeModulation_Control."Set optimal amplitude" zi_OptimizeModulation_Control."Sit Idle"] -> w207
      tunnel: w206 -> [w217 w228 _ w261 w313 w373 w394]
      tunnel: [w216 w227 w237 w261 w313 w374 w393] -> w203
      tunnel: w205 -> [w216 w227 _ w262 w316 w374 w393]
      frame "Sit Idle", Default {
        n83 = event shown="[1] \"Optimize PSHet\": Value Change" {
          selector: _ -> [_ _]
          dyn-events: _ -> [_ _]
          timeout: 5 -> [_ _]
          tunnel: [zi_OptimizeModulation_Control."Sit Idle" w223] -> w221
          event Timeout {
            n84 = event-data() -> ()  [unwired: 1 in, 3 out]
          }
          event "Optimize PSHet": Value Change {
            n85 = event-data() -> ("NewVal"=w226:bool)  [unwired: 1 in]
            n86 = Select(t=zi_OptimizeModulation_Control."Disable PSHet", s=w226, f=zi_OptimizeModulation_Control."Sit Idle") -> (s? t:f=w223:T2)
          }
        }
      }
      frame "Disable PSHet" {
        n87 = flat-sequence {
          frame #0 {
            # "Turn off PSHet first!"
            n88 = local write "Status"("Disabling PSHet..." ("Status")) -> ()
            n89 = property on="Enable PSHet" class="Bool (strict)"("Val(Sgnl)"=FALSE ("Value (Signaling)")) -> ()  [unwired: 2 in, 2 out]
          }
          frame #1 {
            n90 = while "Wait until PSHet is no longer running" {
              stop <- w235 stop-if-true
              n91 = property on="PSHet running" class="Bool (strict)"() -> ("Value"=w236:bool)  [unwired: 2 in, 2 out]
              n92 = Not(x=w236) -> (.not. x?=w235:bool)
            }
          }
        }
      }
      frame "Prepare optimization" {
        w239 = 1
        n93 = Initialize Array(0.0, w239, w239) -> (w242:dbl[][])
        n94 = local read "Starting V"() -> (w243:dbl)
        n95 = local read "Ending V"() -> (w246:dbl)
        n96 = property on="Waveform Chart" class="WFChart (strict)"("History Data"=w242) -> ()  [unwired: 2 in, 2 out]
        n97 = local read "N voltages"() -> (w245:dbl)
        n98 = Subtract(x=w246, y=w243) -> (x-y=w244:dbl)
        n99 = local read "N voltages"() -> (w248:dbl)
        n100 = local write "Status"("Optimizing PSHet...") -> ()
        n101 = Divide(x=w244, y=w245) -> (x/y=w241:dbl)
        n102 = Multiply(x="time", y="Sample rate") -> (x*y=w249:dbl)
        "Samples per acquisition:" <- w249
        n103 = property on="Phase leakage vs. modulation amplitude" class="WFGraph (strict)"("XScale.Multiplier"=w241, "XScale.Offset"=w243) -> ()  [unwired: 2 in, 2 out]
        n104 = Multiply(x=w248, y=w249) -> (x*y=→"Chart length needed:":dbl)
        n105 = Initialize Array(nan, "N voltages") -> (w260:dbl[])
        n106 = call-poly <vilib>:"Ramp Pattern.vi"("start"="Starting V", "end"="Ending V", "samples"="N voltages") -> ("Ramp Pattern"=w237:dbl[])  [unwired: 7 in, 1 out]
      }
      frame "Enable wiggling" {
        w266 = "mods/1/enable"
        # "Turn off mod if\nit was on"
        # "Check if mod was on"
        # "Enable wiggling"
        n107 = local read "Fast wiggler\nsource"() -> (w289:i32)
        n108 = local read "Slow wiggler source"() -> (w265:i32)
        n109 = call-poly <instrlib>:"ziGetValue.vi"("error in"=w299, "Path"=w266, "Handle in"=w300) -> ("error out"=w267:errorcluster, "Value"=w298:dbl, "Handle out"=w270:T4)
        n110 = Decrement(x=w289) -> (x-1=w291:i32)
        n111 = Not Equal To 0?(x=w298) -> (x != 0?=w271:bool)
        n112 = local read "Slow wiggler source"() -> (w284:i32)
        n113 = local write "Keep mod2 activated?"(w271) -> ()
        n114 = case shown="True" w271 {
          tunnel: w270 -> [w306 w312]
          tunnel: [w306 w311] -> w269
          tunnel: [w305 w307] -> w268
          tunnel: w267 -> [w305 w308]
          tunnel: w266 -> [_ w310]
          frame False {
          }
          frame True {
            n115 = call-poly <instrlib>:"ziSetValue.vi"("Error In"=w308, "Value"=0, "Path"=w310, "Handle In"=w312) -> ("Error Out"=w307:errorcluster, "Handle Out"=w311:T4)  [unwired: 1 in]
          }
        }
        n116 = Decrement(x=w265) -> (x-1=w282:i32)
        n117 = Number To Decimal String(number=w291) -> (decimal integer string=w290:string)  [unwired: 1 in]
        n118 = Concatenate Strings("sigouts/0/amplitudes/", w290) -> (w288:string)
        n119 = Number To Decimal String(number=w282) -> (decimal integer string=w281:string)  [unwired: 1 in]
        n120 = local read "Slow wiggler source"() -> (w296:i32)
        n121 = local write "Fast wiggler amp address"(w288) -> ()
        n122 = Decrement(x=w284) -> (x-1=w286:i32)
        n123 = Concatenate Strings("demods/", w281, "/oscselect/") -> (w280:string)
        n124 = Decrement(x=w296) -> (x-1=w295:i32)
        n125 = Decrement(x="Slow wiggler oscillator") -> (x-1=w272:i32)
        n126 = Number To Decimal String(number=w286) -> (decimal integer string=w285:string)  [unwired: 1 in]
        n127 = local write "Slow wiggler osc address"(w280) -> ()
        n128 = call-poly <instrlib>:"ziSetValue.vi"("Error In"=w268, "Value"=w272, "Path"=w280, "Handle In"=w269) -> ("Error Out"=w278:errorcluster, "Handle Out"=w279:T4)  [unwired: 1 in]
        n129 = Concatenate Strings("sigouts/0/amplitudes/", w285) -> (w275:string)
        n130 = Number To Decimal String(number=w295) -> (decimal integer string=w294:string)  [unwired: 1 in]
        n131 = local write "Slow wiggler amp address"(w275) -> ()
        n132 = call-poly <instrlib>:"ziSetValue.vi"("Error In"=w278, "Value"="Slow wiggler amp", "Path"=w275, "Handle In"=w279) -> ("Error Out"=w276:errorcluster, "Handle Out"=w277:T4)  [unwired: 1 in]
        n133 = Concatenate Strings("sigouts/0/enables/", w294) -> (w293:string)
        n134 = local write "Slow wiggler enable address"(w293) -> ()
        n135 = call-poly <instrlib>:"ziSetValue.vi"("Error In"=w276, "Value"=1.0, "Path"=w293, "Handle In"=w277) -> ("Error Out"=w302:errorcluster, "Handle Out"=w304:T4)  [unwired: 1 in]
      }
      frame "Measure phase leakages" {
        n136 = while "While loop: try each AC amplitude and record phase leakage" {
          shift-right: [w332] -> w319
          shift-left: w321 -> [w338]
          shift-right: [w333] -> w320
          shift-left: w318 -> [w337]
          tunnel: w313 -> [w336] mode=indexing
          shift-right: [w327] -> w314
          shift-left: w316 -> [w330]
          i -> [w328]
          stop <- w331 stop-if-true
          # "(0) Set the wiggler amplitude, then (1) do a measurement of phase leakage"
          # "latest phase leakage value"
          n137 = stacked-sequence {
            tunnel: w338 -> [w349 _]
            tunnel: w337 -> [w348 _]
            tunnel: w336 -> [w347 _]
            tunnel: [w342 _] -> w333
            tunnel: [w341 _] -> w332
            tunnel: [_ w358] -> w329
            frame #0 {
              n138 = local read "Fast wiggler amp address"() -> (w340:string)
              n139 = case shown="True" "Update\nmodulation" {
                tunnel: w349 -> [w351 w357]
                tunnel: w348 -> [w350 w356]
                tunnel: w347 -> [_ w355]
                tunnel: [w351 w354] -> w345
                tunnel: [w350 w353] -> w344
                tunnel: w340 -> [_ w352]
                frame False {
                }
                frame True {
                  n140 = call-poly <instrlib>:"ziSetValue.vi"("Error In"=w356, "Value"=w355, "Path"=w352, "Handle In"=w357) -> ("Error Out"=w353:errorcluster, "Handle Out"=w354:T4)  [unwired: 1 in]
                }
              }
              n141 = call-poly <instrlib>:"ziGetValue.vi"("error in"=w344, "Path"=w340, "Handle in"=w345) -> ("error out"=w342:errorcluster, "Value"=→"Present modulation":dbl, "Handle out"=w341:T4)
            }
            frame #1 {
              n142 = local read "Samples per acquisition:"() -> (w363:dbl)
              n143 = local read "Sample rate"() -> (w362:dbl)
              n144 = call "DAQ Assistant"("rate"=w362, "number of samples"=w363) -> ("data"=w368:dynamicdata)  [unwired: 15 in, 2 out]
              n145 = call "Convert from Dynamic Data"("Dynamic Data Type"=w368) -> ("Array"=w367:dbl[][])  [unwired: 3 in]
              n146 = Index Array(array=w367, index (row) #1=1, index (row) #2=0) -> (element #1=w370:dbl[], element #2=w365:dbl[])  [unwired: 2 in]
              n147 = Re/Im To Polar(2:w365, 3:w370) -> (1:w361:dbl[])  [unwired: 1 out]
              n148 = call-poly <vilib>:"TSA Deviation and Variance.vi"("Xt"=w361) -> ("standard deviation"=w360:dbl)  [unwired: 7 in, 3 out]
              n149 = call-poly <vilib>:"TSA Mean.vi"("Xt"=w361) -> ("mean"=w359:dbl)  [unwired: 9 in, 1 out]
              n150 = Build Array (concatenate)(w367, w361) -> (w369:dbl[][])
              n151 = Divide(x=w360, y=w359) -> (x/y=w358:dbl)
              n152 = Transpose 2D Array(2D array=w369) -> (transposed array=→"Waveform Chart":dbl[][])
            }
          }
          n153 = local read "N voltages"() -> (w335:dbl)
          n154 = Decrement(x=w335) -> (x-1=w334:dbl)
          n155 = local read "Stop Program"() -> (w322:bool)
          n156 = Unbundle By Name(w333) -> ("status"=w339:bool)
          n157 = Equal?(x=w328, y=w334) -> (x = y?=w325:bool)
          n158 = Replace Array Subset(array=w330, new element=w329, index=w328) -> (w327:dbl[])
          "Phase leakage vs. modulation amplitude" <- w327
          n159 = Or(x=w339, y=w322) -> (x .or. y?=w326:bool)
          n160 = Or(x=w326, y="Cancel Button") -> (x .or. y?=w324:bool)
          n161 = Or(x=w325, y=w324) -> (x .or. y?=w331:bool)
        }
      }
      frame "Fit phase leakages" {
        n162 = node(w380, w378, "fit_phase_leakage", w379, w374, w374, w373, "Optimization order") -> (w381:refnum<k35>, w377:errorcluster, w382:dbl[])  [unwired: 3 in, 2 out]
        n163 = property on="Phase leakage vs. modulation amplitude" class="WFGraph (strict)"("Value"=w382) -> ()  [unwired: 2 in, 2 out]
      }
      frame "Set optimal amplitude" {
        # "Set optimal modulation amplitude"
        # "Disable slow wiggling"
        n164 = local write "Optimize PSHet"(FALSE) -> ()
        n165 = local read "Fast wiggler amp address"() -> (w396:string)
        n166 = local read "Slow wiggler enable address"() -> (w397:string)
        n167 = node(w406, w407, "get_best_amp", w404, 0.0, w394) -> (w405:refnum<k35>, w401:errorcluster, w395:dbl)  [unwired: 1 in, 2 out]
        "Optimal modulation" <- w395
        n168 = local write "Present modulation"(w395) -> ()
        n169 = call-poly <instrlib>:"ziSetValue.vi"("Error In"=w401, "Value"=w395, "Path"=w396, "Handle In"=w402) -> ("Error Out"=w399:errorcluster, "Handle Out"=w400:T4)  [unwired: 1 in]
        n170 = local read "Keep mod2 activated?"() -> (w390:bool)
        n171 = call-poly <instrlib>:"ziSetValue.vi"("Error In"=w399, "Value"=0.0, "Path"=w397, "Handle In"=w400) -> ("Error Out"=w386:errorcluster, "Handle Out"=w389:T4)  [unwired: 1 in]
        n172 = case "Re-enable Mod2 if it was originally on" shown="True" w390 {
          tunnel: w389 -> [w410 w416]
          tunnel: [w410 w415] -> w388
          tunnel: [w411 w414] -> w387
          tunnel: w386 -> [w411 w413]
          tunnel: [w409 w412] -> w385
          tunnel: TRUE ("Value (Signaling)") -> [w409 w412]
          frame False {
          }
          frame True {
            n173 = call-poly <instrlib>:"ziSetValue.vi"("Error In"=w413, "Value"=1.0, "Path"="mods/1/enable", "Handle In"=w416) -> ("Error Out"=w414:errorcluster, "Handle Out"=w415:T4)  [unwired: 1 in]
          }
        }
        n174 = property on="Enable PSHet" class="Bool (strict)"("Val(Sgnl)"=w385) -> ()  [unwired: 2 in, 2 out]
      }
    }
    n175 = Wait (ms)(milliseconds to wait=5) -> ()  [unwired: 1 out]
    n176 = local write "PSHet Optimization Errors"(w200) -> ()
    n177 = local read "Stop Program"() -> (w211:bool)
  }
  n178 = Close Python Session(session in=w8, error in=w10) -> (11:w11:errorcluster)
  n179 = call <instrlib>:"ziClose.vi"("Error In"=w11, "Handle In"=w9) -> ()  [unwired: 4 out]
